vi "Autonomous Independent.vi"() -> ()   [LabVIEW 2020]
doc: "This VI is called when autonomous begins, and will automatically be terminated when autonomous ends. You can carry out timed or sensor driven robot movement independently without needing to return to the caller."
uses:
  <vilib>/Rock Robotics/WPI/Utilities/WPI_GetSetVariantRefNum.vi
  <vilib>/Rock Robotics/Network Tables/NT Read String.vi
  <vilib>/Rock Robotics/Network Tables/NT Write Numeric Array.vi
  Robot Global Data.vi
  <vilib>/addons/control/pid/pid.llb/PID (DBL).vi
  <vilib>/Rock Robotics/Network Tables/NT Write String.vi
  <vilib>/addons/control/pid/NI_PID_pid.lvlib
panel:
  out "Current action":string
  # "Be sure to right-click and choose Data Operations>>Make Current Value default if you want to save the array values with the VI"
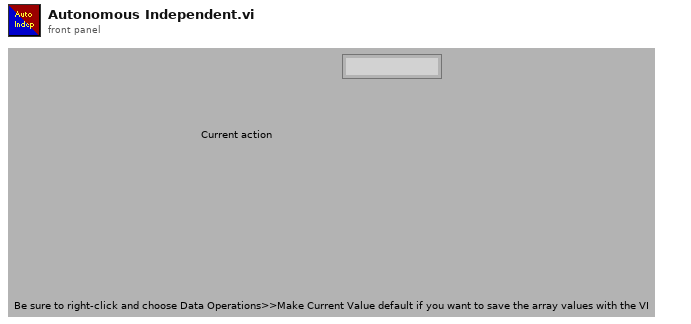
[diagram p1: front panel]
types:
  T1 = typedef "WPI_JoystickDevRef.ctl" = cluster{"Device":T2}
  T2 = typedef "WPI_JoystickDeviceEnum.ctl" = enum16{"USB 0", "USB 1", "USB 2", "USB 3", "USB 4", "USB 5"}
  T3 = cluster{"proportional gain (Kc)":dbl, "integral time (Ti, min)":dbl, "derivative time (Td, min)":dbl}
  T4 = cluster{dbl, "milliseconds to wait":u32, "Name":string}
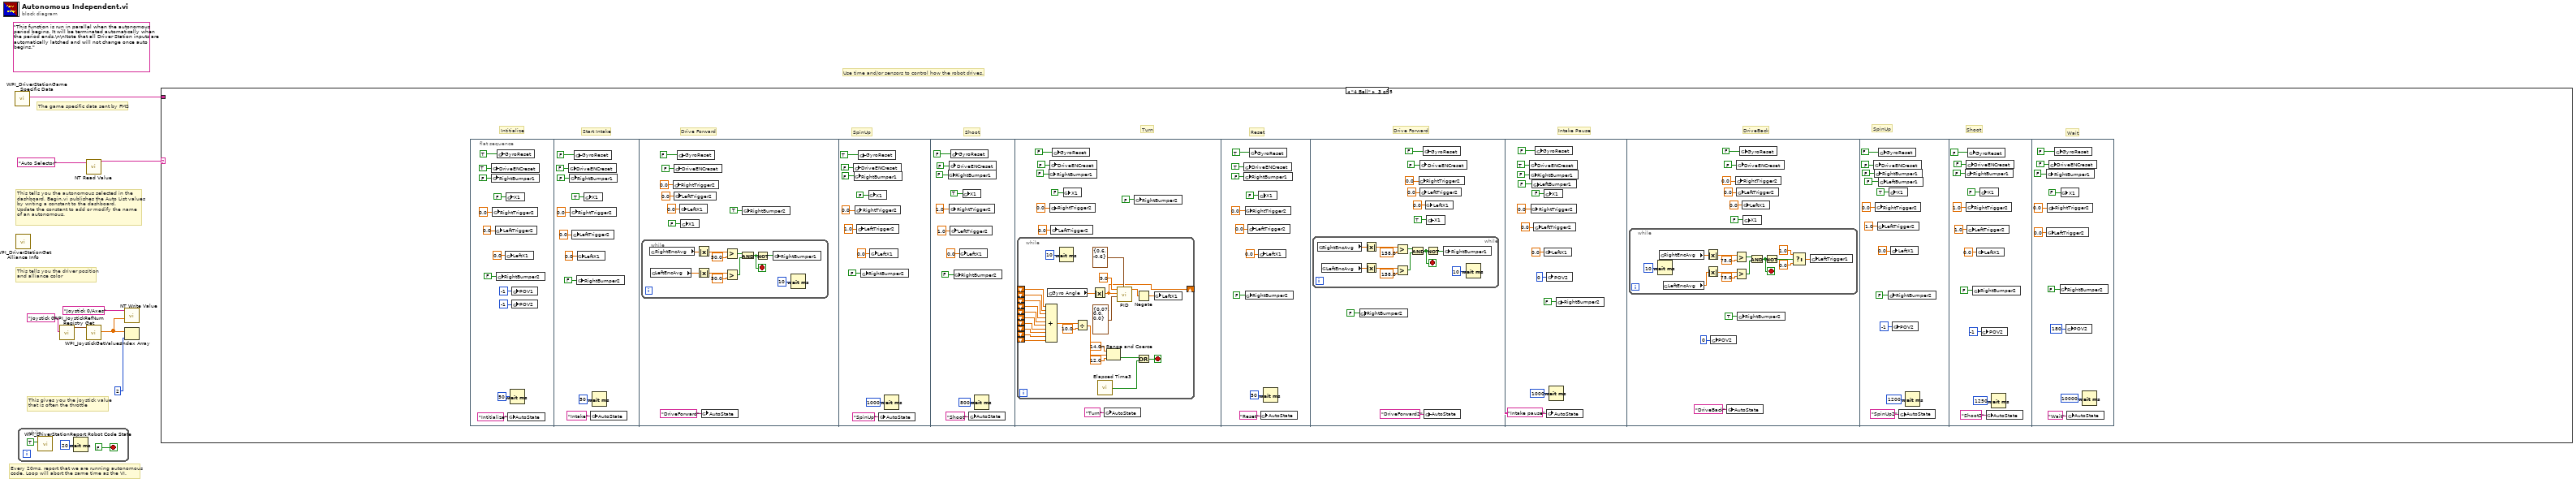
[diagram p0: block diagram]
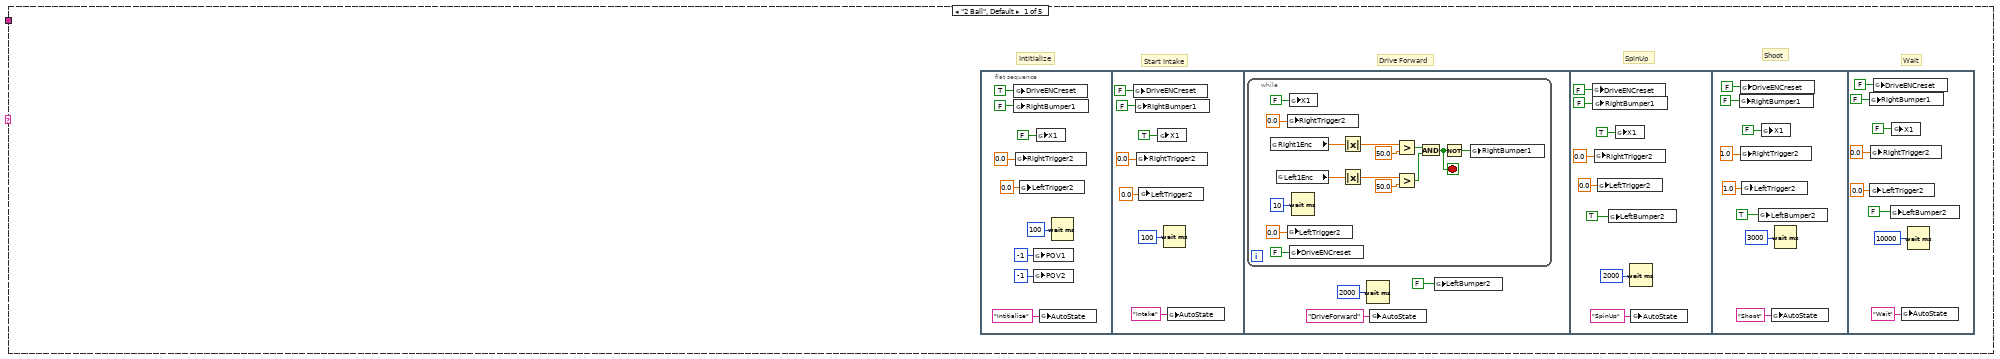
[diagram p2: hidden frame]
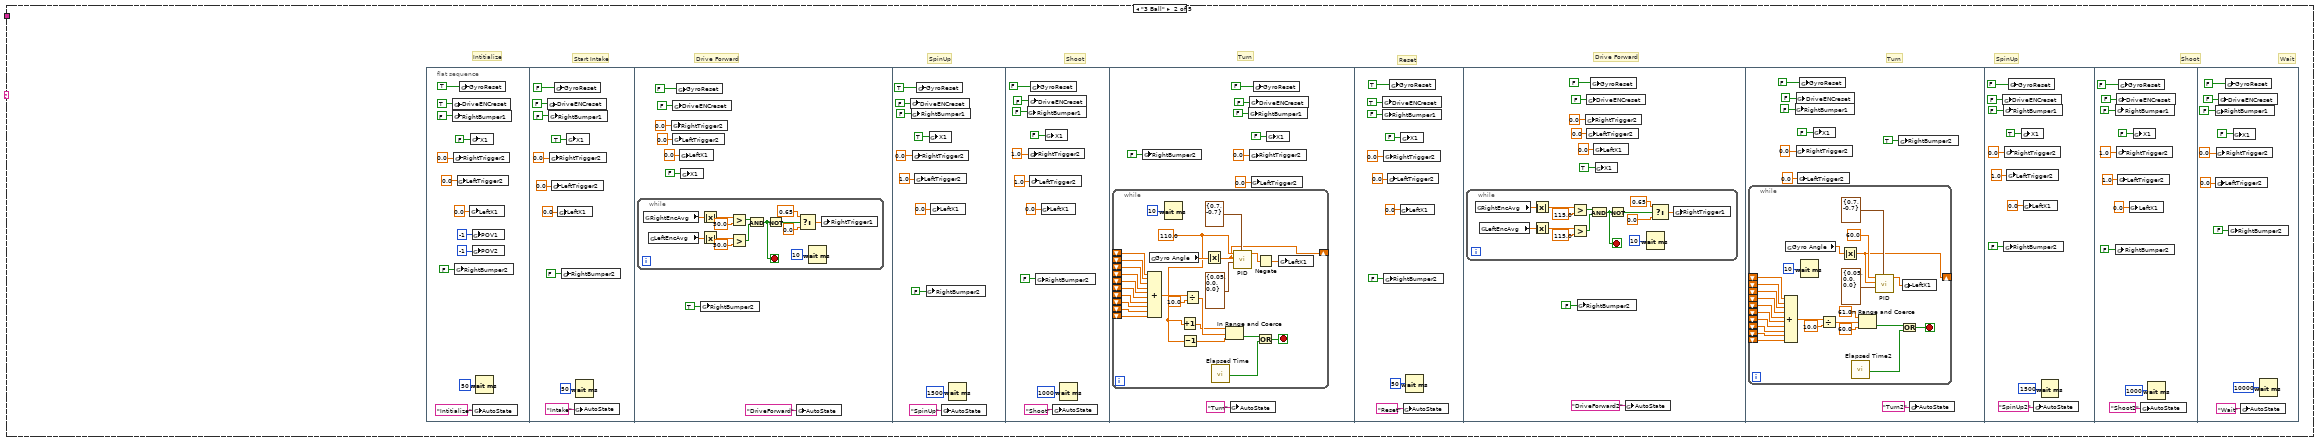
[diagram p3: hidden frame]
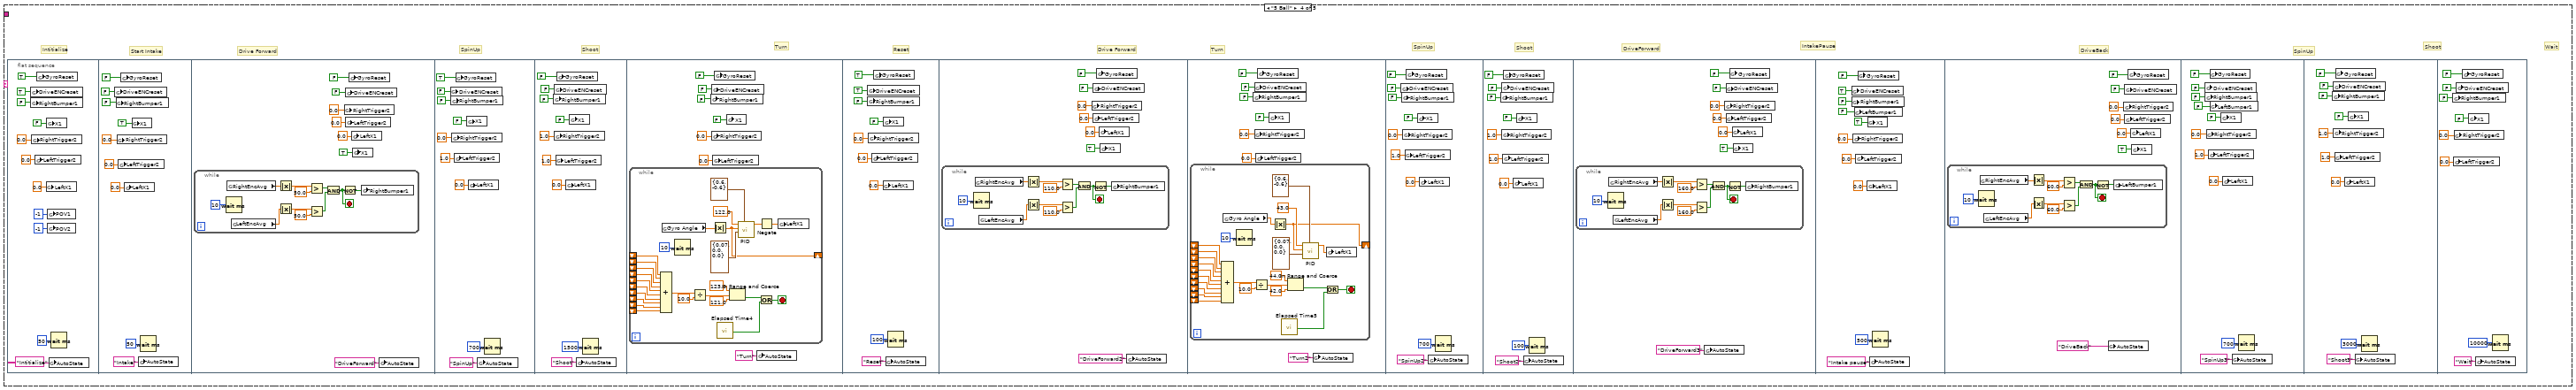
[diagram p4: hidden frame]
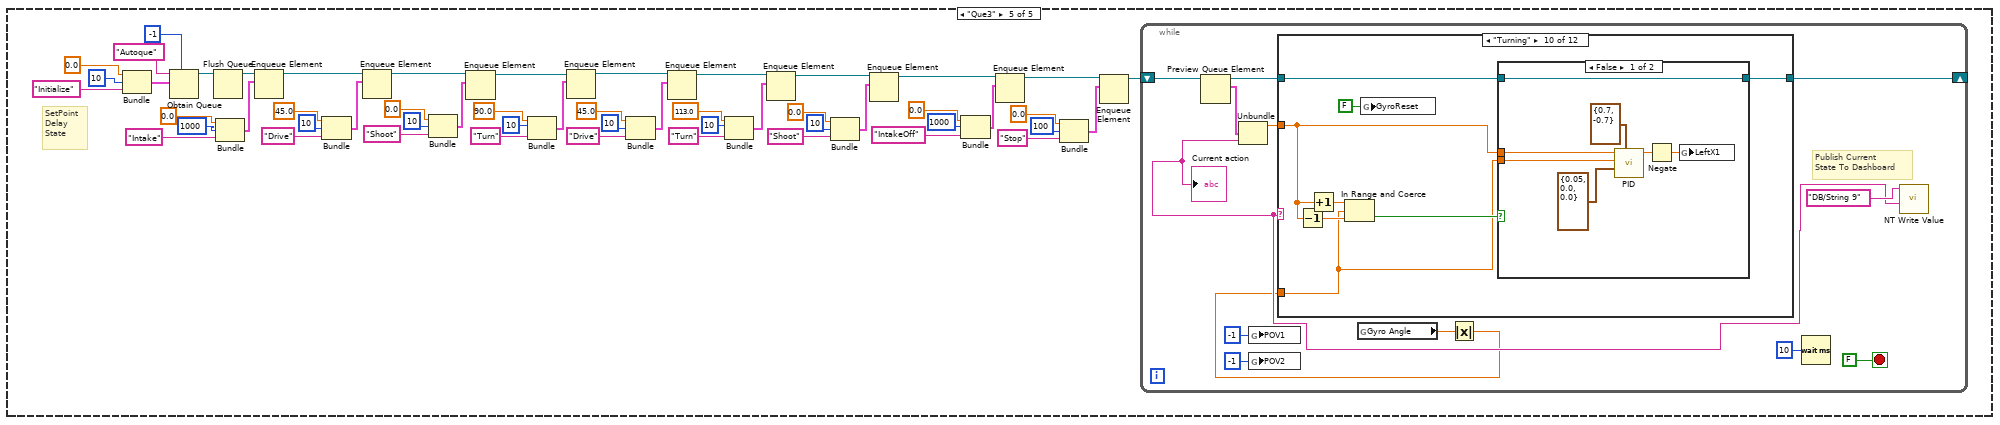
[diagram p5: hidden frame]
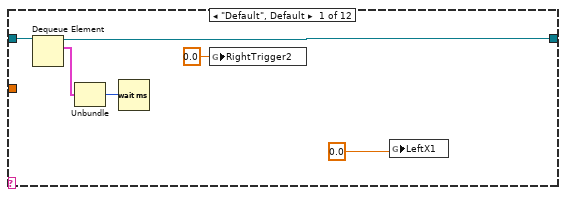
[diagram p6: hidden frame]
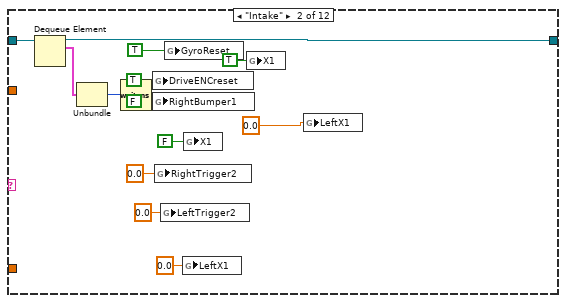
[diagram p7: hidden frame]
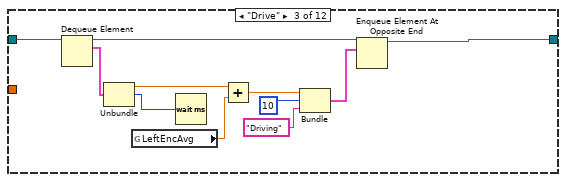
[diagram p8: hidden frame]
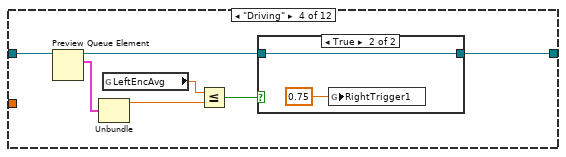
[diagram p9: hidden frame]
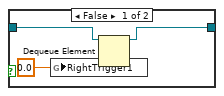
[diagram p10: hidden frame]
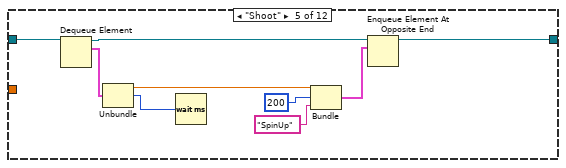
[diagram p11: hidden frame]
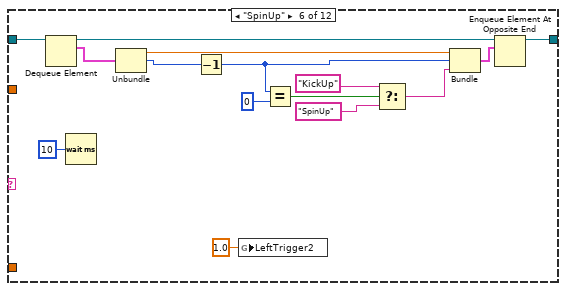
[diagram p12: hidden frame]
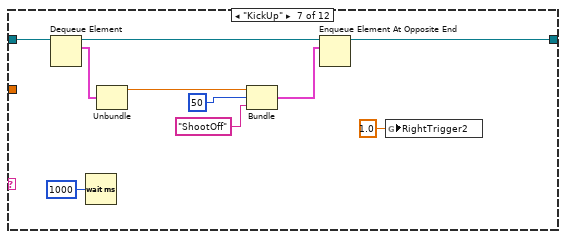
[diagram p13: hidden frame]
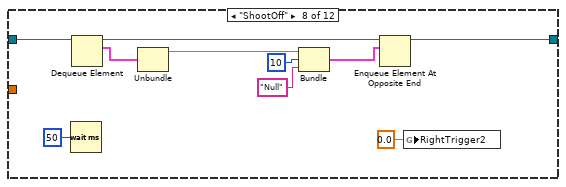
[diagram p14: hidden frame]
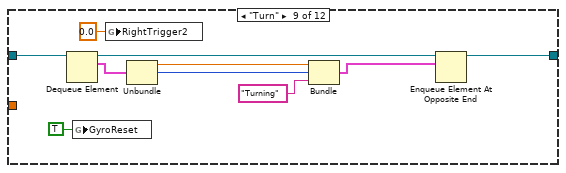
[diagram p15: hidden frame]
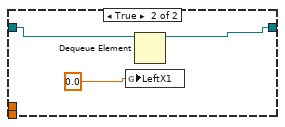
[diagram p16: hidden frame]
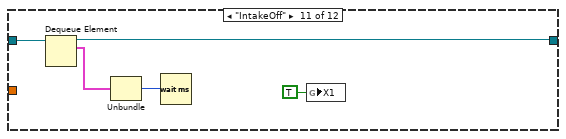
[diagram p17: hidden frame]
diagram:
  (unwired) "This function is run in parallel when the autonomous period begins. It will be terminated automatically when the period ends.\n\nNote that all Driver Station inputs are automatically latched and will not change once auto begins."
  # "The game specific data sent by FMS"
  # "This tells you the autonomous selected in the \ndashboard. Begin.vi publishes the Auto List values\nby writing a constant to the dashboard.\nUpdate the constant to add or modify the name\nof an autonomous."
  # "Every 20ms, report that we are running autonomous\ncode. Loop will abort the same time as the VI."
  # "This gives you the joystick value\nthat is often the throttle"
  # "Use time and/or sensors to control how the robot drives."
  # "This tells you the driver position\nand alliance color"
  n1 = call <vilib>:"WPI_DriverStationGame Specific Data.vi"() -> ("Game Specific Data"=w1:string)  [unwired: 11 in]
  n2 = call <vilib>:"WPI_DriverStationGet Alliance Info.vi"() -> ()  [unwired: 12 out]
  n3 = while {
    stop <- FALSE stop-if-true
    n4 = call <vilib>:"WPI_DriverStationReport Robot Code State.vi"("Autonomous"=TRUE) -> ()  [unwired: 10 in, 1 out]
    n5 = Wait (ms)(milliseconds to wait=u32 20) -> ()  [unwired: 1 out]
  }
  n6 = call <vilib>:"WPI_JoystickRefNum Registry Get.vi"("refnum name"="Joystick 0") -> ("JoystickDevRef"=w7:T1)  [unwired: 1 in, 9 out]
  n7 = call <vilib>:"WPI_JoystickGetValues.vi"("JoystickDevRef"=w7) -> ("Axes"=w3:dbl[])  [unwired: 6 in, 4 out]
  n8 = call-poly <vilib>:"NT Read Value.vi"("Name"="Auto Selector") -> ("String"=w4:string)  [unwired: 9 in, 1 out]
  n9 = call-poly <vilib>:"NT Write Value.vi"("Numeric Array"=w3, "Name"="Joystick 0/Axes") -> ()  [unwired: 9 in, 1 out]
  n10 = Index Array(array=w3, index=2) -> ()  [unwired: 1 out]
  n11 = case shown="\"4 Ball\"" w4 {
    tunnel: w1 -> [_ _ _ _ _]
    frame "2 Ball", Default {
      # "Wait"
      # "Shoot"
      # "SpinUp"
      # "Drive Forward"
      # "Start Intake"
      # "Intitialize"
      n12 = flat-sequence {
        frame #0 {
          n13 = global write "Robot Global Data.vi" "DriveENCreset"(TRUE ("RightBumper1")) -> ()
          n14 = global write "Robot Global Data.vi" "RightBumper1"(FALSE ("RightBumper1")) -> ()
          n15 = global write "Robot Global Data.vi" "RightTrigger2"(0.0 ("RightTrigger2")) -> ()
          n16 = global write "Robot Global Data.vi" "LeftTrigger2"(0.0 ("LeftTrigger2")) -> ()
          n17 = global write "Robot Global Data.vi" "POV1"(i16 -1 ("POV1")) -> ()
          n18 = global write "Robot Global Data.vi" "POV2"(i16 -1 ("POV2")) -> ()
          n19 = global write "Robot Global Data.vi" "X1"(FALSE ("X1")) -> ()
          n20 = global write "Robot Global Data.vi" "AutoState"("Intitialize" ("AutoState")) -> ()
          n21 = Wait (ms)(milliseconds to wait=u32 100) -> ()  [unwired: 1 out]
        }
        frame #1 {
          n22 = global write "Robot Global Data.vi" "DriveENCreset"(FALSE ("RightBumper1")) -> ()
          n23 = global write "Robot Global Data.vi" "RightBumper1"(FALSE ("RightBumper1")) -> ()
          n24 = global write "Robot Global Data.vi" "RightTrigger2"(0.0 ("RightTrigger2")) -> ()
          n25 = global write "Robot Global Data.vi" "LeftTrigger2"(0.0 ("LeftTrigger2")) -> ()
          n26 = global write "Robot Global Data.vi" "X1"(TRUE ("X1")) -> ()
          n27 = Wait (ms)(milliseconds to wait=u32 100) -> ()  [unwired: 1 out]
          n28 = global write "Robot Global Data.vi" "AutoState"("Intake" ("AutoState")) -> ()
        }
        frame #2 {
          n29 = while {
            stop <- w32 stop-if-true
            n30 = global read "Robot Global Data.vi" "Right1Enc"() -> (w43:dbl)
            n31 = global read "Robot Global Data.vi" "Left1Enc"() -> (w42:dbl)
            n32 = global write "Robot Global Data.vi" "RightTrigger2"(0.0 ("RightTrigger2")) -> ()
            n33 = global write "Robot Global Data.vi" "LeftTrigger2"(0.0 ("LeftTrigger2")) -> ()
            n34 = global write "Robot Global Data.vi" "X1"(FALSE ("X1")) -> ()
            n35 = global write "Robot Global Data.vi" "DriveENCreset"(FALSE ("RightBumper1")) -> ()
            n36 = Wait (ms)(milliseconds to wait=u32 10) -> ()  [unwired: 1 out]
            n37 = Absolute Value(x=w43) -> (abs(x)=w35:dbl)
            n38 = Absolute Value(x=w42) -> (abs(x)=w34:dbl)
            n39 = Greater?(x=w35, y=50.0) -> (0:w40:bool)
            n40 = Greater?(x=w34, y=50.0) -> (0:w41:bool)
            n41 = And(x=w40, y=w41) -> (x .and. y?=w32:bool)
            n42 = Not(x=w32) -> (.not. x?=w37:bool)
            n43 = global write "Robot Global Data.vi" "RightBumper1"(w37) -> ()
          }
          n44 = Wait (ms)(milliseconds to wait=u32 2000) -> ()  [unwired: 1 out]
          n45 = global write "Robot Global Data.vi" "AutoState"("DriveForward" ("AutoState")) -> ()
          n46 = global write "Robot Global Data.vi" "LeftBumper2"(FALSE ("RightBumper1")) -> ()
        }
        frame #3 {
          n47 = global write "Robot Global Data.vi" "DriveENCreset"(FALSE ("RightBumper1")) -> ()
          n48 = global write "Robot Global Data.vi" "RightBumper1"(FALSE ("RightBumper1")) -> ()
          n49 = global write "Robot Global Data.vi" "RightTrigger2"(0.0 ("RightTrigger2")) -> ()
          n50 = global write "Robot Global Data.vi" "LeftTrigger2"(0.0 ("LeftTrigger2")) -> ()
          n51 = global write "Robot Global Data.vi" "LeftBumper2"(TRUE ("RightBumper1")) -> ()
          n52 = global write "Robot Global Data.vi" "X1"(TRUE ("X1")) -> ()
          n53 = Wait (ms)(milliseconds to wait=u32 2000) -> ()  [unwired: 1 out]
          n54 = global write "Robot Global Data.vi" "AutoState"("SpinUp" ("AutoState")) -> ()
        }
        frame #4 {
          n55 = global write "Robot Global Data.vi" "RightBumper1"(FALSE ("RightBumper1")) -> ()
          n56 = global write "Robot Global Data.vi" "DriveENCreset"(FALSE ("RightBumper1")) -> ()
          n57 = global write "Robot Global Data.vi" "RightTrigger2"(1.0 ("RightTrigger2")) -> ()
          n58 = global write "Robot Global Data.vi" "LeftTrigger2"(1.0 ("LeftTrigger2")) -> ()
          n59 = global write "Robot Global Data.vi" "LeftBumper2"(TRUE ("RightBumper1")) -> ()
          n60 = global write "Robot Global Data.vi" "X1"(FALSE ("X1")) -> ()
          n61 = global write "Robot Global Data.vi" "AutoState"("Shoot" ("AutoState")) -> ()
          n62 = Wait (ms)(milliseconds to wait=u32 3000) -> ()  [unwired: 1 out]
        }
        frame #5 {
          n63 = global write "Robot Global Data.vi" "RightBumper1"(FALSE ("RightBumper1")) -> ()
          n64 = global write "Robot Global Data.vi" "LeftTrigger2"(0.0 ("LeftTrigger2")) -> ()
          n65 = global write "Robot Global Data.vi" "RightTrigger2"(0.0 ("RightTrigger2")) -> ()
          n66 = global write "Robot Global Data.vi" "DriveENCreset"(FALSE ("RightBumper1")) -> ()
          n67 = global write "Robot Global Data.vi" "LeftBumper2"(FALSE ("RightBumper1")) -> ()
          n68 = global write "Robot Global Data.vi" "X1"(FALSE ("X1")) -> ()
          n69 = global write "Robot Global Data.vi" "AutoState"("Wait" ("AutoState")) -> ()
          n70 = Wait (ms)(milliseconds to wait=u32 10000) -> ()  [unwired: 1 out]
        }
      }
    }
    frame "3 Ball" {
      # "Turn"
      # "Shoot"
      # "SpinUp"
      # "Drive Forward"
      # "Reset"
      # "Turn"
      # "Wait"
      # "Shoot"
      # "SpinUp"
      # "Drive Forward"
      # "Start Intake"
      # "Intitialize"
      n71 = flat-sequence {
        frame #0 {
          n72 = global write "Robot Global Data.vi" "DriveENCreset"(TRUE ("RightBumper1")) -> ()
          n73 = global write "Robot Global Data.vi" "RightBumper1"(FALSE ("RightBumper1")) -> ()
          n74 = global write "Robot Global Data.vi" "RightTrigger2"(0.0 ("RightTrigger2")) -> ()
          n75 = global write "Robot Global Data.vi" "RightBumper2"(FALSE ("RightBumper1")) -> ()
          n76 = global write "Robot Global Data.vi" "LeftTrigger2"(0.0 ("LeftTrigger2")) -> ()
          n77 = global write "Robot Global Data.vi" "GyroReset"(TRUE ("RightBumper1")) -> ()
          n78 = global write "Robot Global Data.vi" "LeftX1"(0.0 ("LeftX1")) -> ()
          n79 = global write "Robot Global Data.vi" "X1"(FALSE ("X1")) -> ()
          n80 = global write "Robot Global Data.vi" "POV1"(i16 -1 ("POV1")) -> ()
          n81 = global write "Robot Global Data.vi" "POV2"(i16 -1 ("POV2")) -> ()
          n82 = global write "Robot Global Data.vi" "AutoState"("Intitialize" ("AutoState")) -> ()
          n83 = Wait (ms)(milliseconds to wait=u32 50) -> ()  [unwired: 1 out]
        }
        frame #1 {
          n84 = global write "Robot Global Data.vi" "DriveENCreset"(FALSE ("RightBumper1")) -> ()
          n85 = global write "Robot Global Data.vi" "RightBumper1"(FALSE ("RightBumper1")) -> ()
          n86 = global write "Robot Global Data.vi" "RightTrigger2"(0.0 ("RightTrigger2")) -> ()
          n87 = global write "Robot Global Data.vi" "LeftTrigger2"(0.0 ("LeftTrigger2")) -> ()
          n88 = global write "Robot Global Data.vi" "GyroReset"(FALSE ("RightBumper1")) -> ()
          n89 = global write "Robot Global Data.vi" "LeftX1"(0.0 ("LeftX1")) -> ()
          n90 = global write "Robot Global Data.vi" "RightBumper2"(FALSE ("RightBumper1")) -> ()
          n91 = global write "Robot Global Data.vi" "X1"(TRUE ("X1")) -> ()
          n92 = global write "Robot Global Data.vi" "AutoState"("Intake" ("AutoState")) -> ()
          n93 = Wait (ms)(milliseconds to wait=u32 50) -> ()  [unwired: 1 out]
        }
        frame #2 {
          n94 = while {
            stop <- w104 stop-if-true
            n95 = global read "Robot Global Data.vi" "RightEncAvg"() -> (w113:dbl)
            n96 = global read "Robot Global Data.vi" "LeftEncAvg"() -> (w112:dbl)
            n97 = Absolute Value(x=w113) -> (abs(x)=w107:dbl)
            n98 = Absolute Value(x=w112) -> (abs(x)=w106:dbl)
            n99 = Greater?(x=w107, y=50.0) -> (0:w110:bool)
            n100 = Greater?(x=w106, y=50.0) -> (0:w111:bool)
            n101 = And(x=w110, y=w111) -> (x .and. y?=w104:bool)
            n102 = Not(x=w104) -> (.not. x?=w103:bool)
            n103 = Select(t=0.65, s=w103, f=0.0) -> (s? t:f=w100:dbl)
            n104 = Wait (ms)(milliseconds to wait=u32 10) -> ()  [unwired: 1 out]
            n105 = global write "Robot Global Data.vi" "RightTrigger1"(w100) -> ()
          }
          n106 = global write "Robot Global Data.vi" "RightTrigger2"(0.0 ("RightTrigger2")) -> ()
          n107 = global write "Robot Global Data.vi" "DriveENCreset"(FALSE ("RightBumper1")) -> ()
          n108 = global write "Robot Global Data.vi" "LeftTrigger2"(0.0 ("LeftTrigger2")) -> ()
          n109 = global write "Robot Global Data.vi" "GyroReset"(FALSE ("RightBumper1")) -> ()
          n110 = global write "Robot Global Data.vi" "LeftX1"(0.0 ("LeftX1")) -> ()
          n111 = global write "Robot Global Data.vi" "X1"(FALSE ("X1")) -> ()
          n112 = global write "Robot Global Data.vi" "RightBumper2"(TRUE ("RightBumper1")) -> ()
          n113 = global write "Robot Global Data.vi" "AutoState"("DriveForward" ("AutoState")) -> ()
        }
        frame #3 {
          n114 = global write "Robot Global Data.vi" "DriveENCreset"(FALSE ("RightBumper1")) -> ()
          n115 = global write "Robot Global Data.vi" "RightBumper1"(FALSE ("RightBumper1")) -> ()
          n116 = global write "Robot Global Data.vi" "RightTrigger2"(0.0 ("RightTrigger2")) -> ()
          n117 = global write "Robot Global Data.vi" "LeftTrigger2"(1.0 ("LeftTrigger2")) -> ()
          n118 = global write "Robot Global Data.vi" "GyroReset"(TRUE ("RightBumper1")) -> ()
          n119 = global write "Robot Global Data.vi" "RightBumper2"(FALSE ("RightBumper1")) -> ()
          n120 = global write "Robot Global Data.vi" "X1"(TRUE ("X1")) -> ()
          n121 = global write "Robot Global Data.vi" "LeftX1"(0.0 ("LeftX1")) -> ()
          n122 = global write "Robot Global Data.vi" "AutoState"("SpinUp" ("AutoState")) -> ()
          n123 = Wait (ms)(milliseconds to wait=u32 1500) -> ()  [unwired: 1 out]
        }
        frame #4 {
          n124 = global write "Robot Global Data.vi" "RightBumper1"(FALSE ("RightBumper1")) -> ()
          n125 = global write "Robot Global Data.vi" "DriveENCreset"(FALSE ("RightBumper1")) -> ()
          n126 = global write "Robot Global Data.vi" "RightTrigger2"(1.0 ("RightTrigger2")) -> ()
          n127 = global write "Robot Global Data.vi" "LeftTrigger2"(1.0 ("LeftTrigger2")) -> ()
          n128 = global write "Robot Global Data.vi" "GyroReset"(FALSE ("RightBumper1")) -> ()
          n129 = global write "Robot Global Data.vi" "RightBumper2"(FALSE ("RightBumper1")) -> ()
          n130 = global write "Robot Global Data.vi" "LeftX1"(0.0 ("LeftX1")) -> ()
          n131 = global write "Robot Global Data.vi" "X1"(FALSE ("X1")) -> ()
          n132 = global write "Robot Global Data.vi" "AutoState"("Shoot" ("AutoState")) -> ()
          n133 = Wait (ms)(milliseconds to wait=u32 1000) -> ()  [unwired: 1 out]
        }
        frame #5 {
          n134 = while {
            shift-right: [w143] -> _
            shift-left: _ -> [w161]
            shift-left: _ -> [w160]
            shift-left: _ -> [w159]
            shift-left: _ -> [w158]
            shift-left: _ -> [w162]
            shift-left: _ -> [w163]
            shift-left: _ -> [w157]
            shift-left: _ -> [w156]
            shift-left: _ -> [w155]
            shift-left: _ -> [w154]
            stop <- w149 stop-if-true
            w144 = 110.0 ("setpoint")
            n135 = Compound Arithmetic op=ADD(w163, w162, w161, w160, w159, w158, w157, w156, w155, w154) -> (w152:dbl)
            n136 = global read "Robot Global Data.vi" "Gyro Angle"() -> (w166:dbl)
            n137 = Wait (ms)(milliseconds to wait=u32 10) -> ()  [unwired: 1 out]
            n138 = Increment(x=w144) -> (x+1=w145:dbl)
            n139 = Decrement(x=w144) -> (x-1=w146:dbl)
            n140 = Divide(x=w152, y=10.0) -> (x/y=w151:dbl)
            n141 = Absolute Value(x=w166) -> (abs(x)=w143:dbl)
            n142 = call "Elapsed Time"() -> ("Time has Elapsed"=w148:bool)  [unwired: 12 in, 7 out]
            n143 = In Range and Coerce(upper limit=w145, x=w151, lower limit=w146) -> (In Range?=w164:bool)  [unwired: 1 out]
            n144 = call-poly <vilib>:"PID.vi"("output range"=cluster{"output high":dbl, "output low":dbl} {"output high"=0.7, "output low"=-0.7}, "PID gains"=T3 {"proportional gain (Kc)"=0.05, "integral time (Ti, min)"=0.0, "derivative time (Td, min)"=0.0}, "process variable"=w143, "setpoint"=w144) -> ("output"=w142:dbl)  [unwired: 6 in, 1 out]
            n145 = Negate(x=w142) -> (-x=w147:dbl)
            n146 = Or(x=w164, y=w148) -> (x .or. y?=w149:bool)
            n147 = global write "Robot Global Data.vi" "LeftX1"(w147) -> ()
          }
          n148 = global write "Robot Global Data.vi" "RightBumper2"(FALSE ("RightBumper1")) -> ()
          n149 = global write "Robot Global Data.vi" "AutoState"("Turn" ("AutoState")) -> ()
          n150 = global write "Robot Global Data.vi" "RightBumper1"(FALSE ("RightBumper1")) -> ()
          n151 = global write "Robot Global Data.vi" "DriveENCreset"(FALSE ("RightBumper1")) -> ()
          n152 = global write "Robot Global Data.vi" "RightTrigger2"(0.0 ("RightTrigger2")) -> ()
          n153 = global write "Robot Global Data.vi" "LeftTrigger2"(0.0 ("LeftTrigger2")) -> ()
          n154 = global write "Robot Global Data.vi" "GyroReset"(FALSE ("RightBumper1")) -> ()
          n155 = global write "Robot Global Data.vi" "X1"(FALSE ("X1")) -> ()
        }
        frame #6 {
          n156 = global write "Robot Global Data.vi" "DriveENCreset"(TRUE ("RightBumper1")) -> ()
          n157 = global write "Robot Global Data.vi" "RightBumper1"(FALSE ("RightBumper1")) -> ()
          n158 = global write "Robot Global Data.vi" "RightTrigger2"(0.0 ("RightTrigger2")) -> ()
          n159 = global write "Robot Global Data.vi" "RightBumper2"(FALSE ("RightBumper1")) -> ()
          n160 = global write "Robot Global Data.vi" "LeftTrigger2"(0.0 ("LeftTrigger2")) -> ()
          n161 = global write "Robot Global Data.vi" "GyroReset"(TRUE ("RightBumper1")) -> ()
          n162 = global write "Robot Global Data.vi" "LeftX1"(0.0 ("LeftX1")) -> ()
          n163 = global write "Robot Global Data.vi" "X1"(FALSE ("X1")) -> ()
          n164 = global write "Robot Global Data.vi" "AutoState"("Reset" ("AutoState")) -> ()
          n165 = Wait (ms)(milliseconds to wait=u32 50) -> ()  [unwired: 1 out]
        }
        frame #7 {
          n166 = while {
            stop <- w190 stop-if-true
            n167 = global read "Robot Global Data.vi" "RightEncAvg"() -> (w199:dbl)
            n168 = global read "Robot Global Data.vi" "LeftEncAvg"() -> (w198:dbl)
            n169 = Absolute Value(x=w199) -> (abs(x)=w193:dbl)
            n170 = Absolute Value(x=w198) -> (abs(x)=w192:dbl)
            n171 = Greater?(x=w193, y=115.0) -> (0:w196:bool)
            n172 = Greater?(x=w192, y=115.0) -> (0:w197:bool)
            n173 = And(x=w196, y=w197) -> (x .and. y?=w190:bool)
            n174 = Not(x=w190) -> (.not. x?=w189:bool)
            n175 = Wait (ms)(milliseconds to wait=u32 10) -> ()  [unwired: 1 out]
            n176 = Select(t=0.65, s=w189, f=0.0) -> (s? t:f=w188:dbl)
            n177 = global write "Robot Global Data.vi" "RightTrigger1"(w188) -> ()
          }
          n178 = global write "Robot Global Data.vi" "RightBumper2"(FALSE ("RightBumper1")) -> ()
          n179 = global write "Robot Global Data.vi" "RightTrigger2"(0.0 ("RightTrigger2")) -> ()
          n180 = global write "Robot Global Data.vi" "DriveENCreset"(FALSE ("RightBumper1")) -> ()
          n181 = global write "Robot Global Data.vi" "LeftTrigger2"(0.0 ("LeftTrigger2")) -> ()
          n182 = global write "Robot Global Data.vi" "GyroReset"(FALSE ("RightBumper1")) -> ()
          n183 = global write "Robot Global Data.vi" "LeftX1"(0.0 ("LeftX1")) -> ()
          n184 = global write "Robot Global Data.vi" "X1"(TRUE ("X1")) -> ()
          n185 = global write "Robot Global Data.vi" "AutoState"("DriveForward2" ("AutoState")) -> ()
        }
        frame #8 {
          n186 = while {
            shift-right: [w208] -> _
            shift-left: _ -> [w222]
            shift-left: _ -> [w221]
            shift-left: _ -> [w220]
            shift-left: _ -> [w219]
            shift-left: _ -> [w223]
            shift-left: _ -> [w224]
            shift-left: _ -> [w218]
            shift-left: _ -> [w217]
            shift-left: _ -> [w216]
            shift-left: _ -> [w215]
            stop <- w210 stop-if-true
            n187 = Compound Arithmetic op=ADD(w224, w223, w222, w221, w220, w219, w218, w217, w216, w215) -> (w213:dbl)
            n188 = global read "Robot Global Data.vi" "Gyro Angle"() -> (w231:dbl)
            n189 = Wait (ms)(milliseconds to wait=u32 10) -> ()  [unwired: 1 out]
            n190 = Divide(x=w213, y=10.0) -> (x/y=w212:dbl)
            n191 = Absolute Value(x=w231) -> (abs(x)=w208:dbl)
            n192 = call "Elapsed Time2"() -> ("Time has Elapsed"=w209:bool)  [unwired: 12 in, 7 out]
            n193 = In Range and Coerce(upper limit=61.0, x=w212, lower limit=60.0) -> (In Range?=w228:bool)  [unwired: 1 out]
            n194 = call-poly <vilib>:"PID.vi"("output range"=cluster{"output high":dbl, "output low":dbl} {"output high"=0.7, "output low"=-0.7}, "PID gains"=T3 {"proportional gain (Kc)"=0.05, "integral time (Ti, min)"=0.0, "derivative time (Td, min)"=0.0}, "process variable"=w208, "setpoint"=60.0) -> ("output"=w225:dbl)  [unwired: 6 in, 1 out]
            n195 = Or(x=w228, y=w209) -> (x .or. y?=w210:bool)
            n196 = global write "Robot Global Data.vi" "LeftX1"(w225) -> ()
          }
          n197 = global write "Robot Global Data.vi" "RightBumper1"(FALSE ("RightBumper1")) -> ()
          n198 = global write "Robot Global Data.vi" "DriveENCreset"(FALSE ("RightBumper1")) -> ()
          n199 = global write "Robot Global Data.vi" "RightTrigger2"(0.0 ("RightTrigger2")) -> ()
          n200 = global write "Robot Global Data.vi" "LeftTrigger2"(0.0 ("LeftTrigger2")) -> ()
          n201 = global write "Robot Global Data.vi" "GyroReset"(FALSE ("RightBumper1")) -> ()
          n202 = global write "Robot Global Data.vi" "X1"(FALSE ("X1")) -> ()
          n203 = global write "Robot Global Data.vi" "RightBumper2"(TRUE ("RightBumper1")) -> ()
          n204 = global write "Robot Global Data.vi" "AutoState"("Turn2" ("AutoState")) -> ()
        }
        frame #9 {
          n205 = global write "Robot Global Data.vi" "DriveENCreset"(FALSE ("RightBumper1")) -> ()
          n206 = global write "Robot Global Data.vi" "RightBumper1"(FALSE ("RightBumper1")) -> ()
          n207 = global write "Robot Global Data.vi" "RightBumper2"(FALSE ("RightBumper1")) -> ()
          n208 = global write "Robot Global Data.vi" "RightTrigger2"(0.0 ("RightTrigger2")) -> ()
          n209 = global write "Robot Global Data.vi" "LeftTrigger2"(1.0 ("LeftTrigger2")) -> ()
          n210 = global write "Robot Global Data.vi" "GyroReset"(FALSE ("RightBumper1")) -> ()
          n211 = global write "Robot Global Data.vi" "X1"(TRUE ("X1")) -> ()
          n212 = global write "Robot Global Data.vi" "LeftX1"(0.0 ("LeftX1")) -> ()
          n213 = global write "Robot Global Data.vi" "AutoState"("SpinUp2" ("AutoState")) -> ()
          n214 = Wait (ms)(milliseconds to wait=u32 1500) -> ()  [unwired: 1 out]
        }
        frame #10 {
          n215 = global write "Robot Global Data.vi" "RightBumper1"(FALSE ("RightBumper1")) -> ()
          n216 = global write "Robot Global Data.vi" "RightBumper2"(FALSE ("RightBumper1")) -> ()
          n217 = global write "Robot Global Data.vi" "DriveENCreset"(FALSE ("RightBumper1")) -> ()
          n218 = global write "Robot Global Data.vi" "RightTrigger2"(1.0 ("RightTrigger2")) -> ()
          n219 = global write "Robot Global Data.vi" "LeftTrigger2"(1.0 ("LeftTrigger2")) -> ()
          n220 = global write "Robot Global Data.vi" "GyroReset"(FALSE ("RightBumper1")) -> ()
          n221 = global write "Robot Global Data.vi" "LeftX1"(0.0 ("LeftX1")) -> ()
          n222 = global write "Robot Global Data.vi" "X1"(FALSE ("X1")) -> ()
          n223 = global write "Robot Global Data.vi" "AutoState"("Shoot2" ("AutoState")) -> ()
          n224 = Wait (ms)(milliseconds to wait=u32 1000) -> ()  [unwired: 1 out]
        }
        frame #11 {
          n225 = global write "Robot Global Data.vi" "RightBumper1"(FALSE ("RightBumper1")) -> ()
          n226 = global write "Robot Global Data.vi" "LeftTrigger2"(0.0 ("LeftTrigger2")) -> ()
          n227 = global write "Robot Global Data.vi" "RightTrigger2"(0.0 ("RightTrigger2")) -> ()
          n228 = global write "Robot Global Data.vi" "DriveENCreset"(FALSE ("RightBumper1")) -> ()
          n229 = global write "Robot Global Data.vi" "GyroReset"(FALSE ("RightBumper1")) -> ()
          n230 = global write "Robot Global Data.vi" "RightBumper2"(FALSE ("RightBumper1")) -> ()
          n231 = global write "Robot Global Data.vi" "X1"(FALSE ("X1")) -> ()
          n232 = global write "Robot Global Data.vi" "AutoState"("Wait" ("AutoState")) -> ()
          n233 = Wait (ms)(milliseconds to wait=u32 10000) -> ()  [unwired: 1 out]
        }
      }
    }
    frame "4 Ball" {
      # "Intake Pause"
      # "DriveBack"
      # "Shoot"
      # "SpinUp"
      # "Drive Forward"
      # "Reset"
      # "Turn"
      # "Wait"
      # "Shoot"
      # "SpinUp"
      # "Drive Forward"
      # "Start Intake"
      # "Intitialize"
      n234 = flat-sequence {
        frame #0 {
          n235 = global write "Robot Global Data.vi" "DriveENCreset"(TRUE ("RightBumper1")) -> ()
          n236 = global write "Robot Global Data.vi" "RightBumper1"(FALSE ("RightBumper1")) -> ()
          n237 = global write "Robot Global Data.vi" "RightTrigger2"(0.0 ("RightTrigger2")) -> ()
          n238 = global write "Robot Global Data.vi" "LeftTrigger2"(0.0 ("LeftTrigger2")) -> ()
          n239 = global write "Robot Global Data.vi" "RightBumper2"(FALSE ("RightBumper1")) -> ()
          n240 = global write "Robot Global Data.vi" "GyroReset"(TRUE ("RightBumper1")) -> ()
          n241 = global write "Robot Global Data.vi" "LeftX1"(0.0 ("LeftX1")) -> ()
          n242 = global write "Robot Global Data.vi" "X1"(FALSE ("X1")) -> ()
          n243 = global write "Robot Global Data.vi" "AutoState"("Intitialize" ("AutoState")) -> ()
          n244 = Wait (ms)(milliseconds to wait=u32 50) -> ()  [unwired: 1 out]
          n245 = global write "Robot Global Data.vi" "POV1"(i16 -1 ("POV1")) -> ()
          n246 = global write "Robot Global Data.vi" "POV2"(i16 -1 ("POV2")) -> ()
        }
        frame #1 {
          n247 = global write "Robot Global Data.vi" "DriveENCreset"(FALSE ("RightBumper1")) -> ()
          n248 = global write "Robot Global Data.vi" "RightBumper1"(FALSE ("RightBumper1")) -> ()
          n249 = global write "Robot Global Data.vi" "RightTrigger2"(0.0 ("RightTrigger2")) -> ()
          n250 = global write "Robot Global Data.vi" "LeftTrigger2"(0.0 ("LeftTrigger2")) -> ()
          n251 = global write "Robot Global Data.vi" "GyroReset"(FALSE ("RightBumper1")) -> ()
          n252 = global write "Robot Global Data.vi" "RightBumper2"(FALSE ("RightBumper1")) -> ()
          n253 = global write "Robot Global Data.vi" "LeftX1"(0.0 ("LeftX1")) -> ()
          n254 = global write "Robot Global Data.vi" "X1"(TRUE ("X1")) -> ()
          n255 = global write "Robot Global Data.vi" "AutoState"("Intake" ("AutoState")) -> ()
          n256 = Wait (ms)(milliseconds to wait=u32 50) -> ()  [unwired: 1 out]
        }
        frame #2 {
          n257 = while {
            stop <- w292 stop-if-true
            n258 = global read "Robot Global Data.vi" "RightEncAvg"() -> (w302:dbl)
            n259 = global read "Robot Global Data.vi" "LeftEncAvg"() -> (w301:dbl)
            n260 = Absolute Value(x=w302) -> (abs(x)=w295:dbl)
            n261 = Absolute Value(x=w301) -> (abs(x)=w294:dbl)
            n262 = Greater?(x=w295, y=50.0) -> (0:w299:bool)
            n263 = Greater?(x=w294, y=50.0) -> (0:w300:bool)
            n264 = And(x=w299, y=w300) -> (x .and. y?=w292:bool)
            n265 = Not(x=w292) -> (.not. x?=w296:bool)
            n266 = global write "Robot Global Data.vi" "RightBumper1"(w296) -> ()
            n267 = Wait (ms)(milliseconds to wait=u32 10) -> ()  [unwired: 1 out]
          }
          n268 = global write "Robot Global Data.vi" "RightTrigger2"(0.0 ("RightTrigger2")) -> ()
          n269 = global write "Robot Global Data.vi" "DriveENCreset"(FALSE ("RightBumper1")) -> ()
          n270 = global write "Robot Global Data.vi" "LeftTrigger2"(0.0 ("LeftTrigger2")) -> ()
          n271 = global write "Robot Global Data.vi" "GyroReset"(FALSE ("RightBumper1")) -> ()
          n272 = global write "Robot Global Data.vi" "LeftX1"(0.0 ("LeftX1")) -> ()
          n273 = global write "Robot Global Data.vi" "X1"(FALSE ("X1")) -> ()
          n274 = global write "Robot Global Data.vi" "AutoState"("DriveForward" ("AutoState")) -> ()
          n275 = global write "Robot Global Data.vi" "RightBumper2"(TRUE ("RightBumper1")) -> ()
        }
        frame #3 {
          n276 = global write "Robot Global Data.vi" "DriveENCreset"(FALSE ("RightBumper1")) -> ()
          n277 = global write "Robot Global Data.vi" "RightBumper1"(FALSE ("RightBumper1")) -> ()
          n278 = global write "Robot Global Data.vi" "RightTrigger2"(0.0 ("RightTrigger2")) -> ()
          n279 = global write "Robot Global Data.vi" "LeftTrigger2"(1.0 ("LeftTrigger2")) -> ()
          n280 = global write "Robot Global Data.vi" "GyroReset"(TRUE ("RightBumper1")) -> ()
          n281 = global write "Robot Global Data.vi" "RightBumper2"(FALSE ("RightBumper1")) -> ()
          n282 = global write "Robot Global Data.vi" "X1"(FALSE ("X1")) -> ()
          n283 = global write "Robot Global Data.vi" "LeftX1"(0.0 ("LeftX1")) -> ()
          n284 = global write "Robot Global Data.vi" "AutoState"("SpinUp" ("AutoState")) -> ()
          n285 = Wait (ms)(milliseconds to wait=u32 1000) -> ()  [unwired: 1 out]
        }
        frame #4 {
          n286 = global write "Robot Global Data.vi" "RightBumper1"(FALSE ("RightBumper1")) -> ()
          n287 = global write "Robot Global Data.vi" "DriveENCreset"(FALSE ("RightBumper1")) -> ()
          n288 = global write "Robot Global Data.vi" "RightTrigger2"(1.0 ("RightTrigger2")) -> ()
          n289 = global write "Robot Global Data.vi" "LeftTrigger2"(1.0 ("LeftTrigger2")) -> ()
          n290 = global write "Robot Global Data.vi" "GyroReset"(FALSE ("RightBumper1")) -> ()
          n291 = global write "Robot Global Data.vi" "RightBumper2"(FALSE ("RightBumper1")) -> ()
          n292 = global write "Robot Global Data.vi" "LeftX1"(0.0 ("LeftX1")) -> ()
          n293 = global write "Robot Global Data.vi" "X1"(TRUE ("X1")) -> ()
          n294 = global write "Robot Global Data.vi" "AutoState"("Shoot" ("AutoState")) -> ()
          n295 = Wait (ms)(milliseconds to wait=u32 800) -> ()  [unwired: 1 out]
        }
        frame #5 {
          n296 = while {
            shift-right: [w331] -> _
            shift-left: _ -> [w346]
            shift-left: _ -> [w345]
            shift-left: _ -> [w344]
            shift-left: _ -> [w343]
            shift-left: _ -> [w347]
            shift-left: _ -> [w348]
            shift-left: _ -> [w342]
            shift-left: _ -> [w341]
            shift-left: _ -> [w340]
            shift-left: _ -> [w339]
            stop <- w334 stop-if-true
            n297 = Compound Arithmetic op=ADD(w348, w347, w346, w345, w344, w343, w342, w341, w340, w339) -> (w337:dbl)
            n298 = global read "Robot Global Data.vi" "Gyro Angle"() -> (w355:dbl)
            n299 = Wait (ms)(milliseconds to wait=u32 10) -> ()  [unwired: 1 out]
            n300 = Divide(x=w337, y=10.0) -> (x/y=w336:dbl)
            n301 = Absolute Value(x=w355) -> (abs(x)=w331:dbl)
            n302 = call "Elapsed Time3"() -> ("Time has Elapsed"=w333:bool)  [unwired: 12 in, 7 out]
            n303 = In Range and Coerce(upper limit=14.0, x=w336, lower limit=12.0) -> (In Range?=w352:bool)  [unwired: 1 out]
            n304 = call-poly <vilib>:"PID.vi"("output range"=cluster{"output high":dbl, "output low":dbl} {"output high"=0.6, "output low"=-0.6}, "PID gains"=T3 {"proportional gain (Kc)"=0.07, "integral time (Ti, min)"=0.0, "derivative time (Td, min)"=0.0}, "process variable"=w331, "setpoint"=9.0) -> ("output"=w349:dbl)  [unwired: 6 in, 1 out]
            n305 = Negate(x=w349) -> (-x=w332:dbl)
            n306 = Or(x=w352, y=w333) -> (x .or. y?=w334:bool)
            n307 = global write "Robot Global Data.vi" "LeftX1"(w332) -> ()
          }
          n308 = global write "Robot Global Data.vi" "RightBumper1"(FALSE ("RightBumper1")) -> ()
          n309 = global write "Robot Global Data.vi" "DriveENCreset"(FALSE ("RightBumper1")) -> ()
          n310 = global write "Robot Global Data.vi" "RightTrigger2"(0.0 ("RightTrigger2")) -> ()
          n311 = global write "Robot Global Data.vi" "LeftTrigger2"(0.0 ("LeftTrigger2")) -> ()
          n312 = global write "Robot Global Data.vi" "GyroReset"(FALSE ("RightBumper1")) -> ()
          n313 = global write "Robot Global Data.vi" "X1"(FALSE ("X1")) -> ()
          n314 = global write "Robot Global Data.vi" "AutoState"("Turn" ("AutoState")) -> ()
          n315 = global write "Robot Global Data.vi" "RightBumper2"(FALSE ("RightBumper1")) -> ()
        }
        frame #6 {
          n316 = global write "Robot Global Data.vi" "DriveENCreset"(TRUE ("RightBumper1")) -> ()
          n317 = global write "Robot Global Data.vi" "RightBumper1"(FALSE ("RightBumper1")) -> ()
          n318 = global write "Robot Global Data.vi" "RightTrigger2"(0.0 ("RightTrigger2")) -> ()
          n319 = global write "Robot Global Data.vi" "RightBumper2"(FALSE ("RightBumper1")) -> ()
          n320 = global write "Robot Global Data.vi" "LeftTrigger2"(0.0 ("LeftTrigger2")) -> ()
          n321 = global write "Robot Global Data.vi" "GyroReset"(TRUE ("RightBumper1")) -> ()
          n322 = global write "Robot Global Data.vi" "LeftX1"(0.0 ("LeftX1")) -> ()
          n323 = global write "Robot Global Data.vi" "X1"(FALSE ("X1")) -> ()
          n324 = global write "Robot Global Data.vi" "AutoState"("Reset" ("AutoState")) -> ()
          n325 = Wait (ms)(milliseconds to wait=u32 50) -> ()  [unwired: 1 out]
        }
        frame #7 {
          n326 = while {
            stop <- w375 stop-if-true
            n327 = global read "Robot Global Data.vi" "RightEncAvg"() -> (w385:dbl)
            n328 = global read "Robot Global Data.vi" "LeftEncAvg"() -> (w384:dbl)
            n329 = Absolute Value(x=w385) -> (abs(x)=w378:dbl)
            n330 = Absolute Value(x=w384) -> (abs(x)=w377:dbl)
            n331 = Greater?(x=w378, y=158.0) -> (0:w382:bool)
            n332 = Greater?(x=w377, y=158.0) -> (0:w383:bool)
            n333 = And(x=w382, y=w383) -> (x .and. y?=w375:bool)
            n334 = Not(x=w375) -> (.not. x?=w379:bool)
            n335 = global write "Robot Global Data.vi" "RightBumper1"(w379) -> ()
            n336 = Wait (ms)(milliseconds to wait=u32 10) -> ()  [unwired: 1 out]
          }
          n337 = global write "Robot Global Data.vi" "RightBumper2"(FALSE ("RightBumper1")) -> ()
          n338 = global write "Robot Global Data.vi" "RightTrigger2"(0.0 ("RightTrigger2")) -> ()
          n339 = global write "Robot Global Data.vi" "DriveENCreset"(FALSE ("RightBumper1")) -> ()
          n340 = global write "Robot Global Data.vi" "LeftTrigger2"(0.0 ("LeftTrigger2")) -> ()
          n341 = global write "Robot Global Data.vi" "GyroReset"(FALSE ("RightBumper1")) -> ()
          n342 = global write "Robot Global Data.vi" "AutoState"("DriveForward2" ("AutoState")) -> ()
          n343 = global write "Robot Global Data.vi" "LeftX1"(0.0 ("LeftX1")) -> ()
          n344 = global write "Robot Global Data.vi" "X1"(TRUE ("X1")) -> ()
        }
        frame #8 {
          n345 = global write "Robot Global Data.vi" "DriveENCreset"(TRUE ("RightBumper1")) -> ()
          n346 = global write "Robot Global Data.vi" "RightBumper1"(FALSE ("RightBumper1")) -> ()
          n347 = global write "Robot Global Data.vi" "RightTrigger2"(0.0 ("RightTrigger2")) -> ()
          n348 = global write "Robot Global Data.vi" "LeftBumper1"(FALSE ("RightBumper1")) -> ()
          n349 = global write "Robot Global Data.vi" "LeftTrigger2"(0.0 ("LeftTrigger2")) -> ()
          n350 = global write "Robot Global Data.vi" "GyroReset"(FALSE ("RightBumper1")) -> ()
          n351 = global write "Robot Global Data.vi" "LeftX1"(0.0 ("LeftX1")) -> ()
          n352 = global write "Robot Global Data.vi" "X1"(FALSE ("X1")) -> ()
          n353 = global write "Robot Global Data.vi" "POV2"(i16 0 ("POV2")) -> ()
          n354 = global write "Robot Global Data.vi" "AutoState"("Intake pause" ("AutoState")) -> ()
          n355 = Wait (ms)(milliseconds to wait=u32 1000) -> ()  [unwired: 1 out]
          n356 = global write "Robot Global Data.vi" "RightBumper2"(FALSE ("RightBumper1")) -> ()
        }
        frame #9 {
          n357 = while {
            stop <- w411 stop-if-true
            n358 = Wait (ms)(milliseconds to wait=u32 10) -> ()  [unwired: 1 out]
            n359 = global read "Robot Global Data.vi" "RightEncAvg"() -> (w420:dbl)
            n360 = global read "Robot Global Data.vi" "LeftEncAvg"() -> (w419:dbl)
            n361 = Absolute Value(x=w420) -> (abs(x)=w414:dbl)
            n362 = Absolute Value(x=w419) -> (abs(x)=w413:dbl)
            n363 = Greater?(x=w414, y=75.0) -> (0:w417:bool)
            n364 = Greater?(x=w413, y=75.0) -> (0:w418:bool)
            n365 = And(x=w417, y=w418) -> (x .and. y?=w411:bool)
            n366 = Not(x=w411) -> (.not. x?=w410:bool)
            n367 = Select(t=1.0, s=w410, f=0.0) -> (s? t:f=w409:dbl)
            n368 = global write "Robot Global Data.vi" "LeftTrigger1"(w409) -> ()
          }
          n369 = global write "Robot Global Data.vi" "POV2"(i16 0 ("POV2")) -> ()
          n370 = global write "Robot Global Data.vi" "AutoState"("DriveBack" ("AutoState")) -> ()
          n371 = global write "Robot Global Data.vi" "RightTrigger2"(0.0 ("RightTrigger2")) -> ()
          n372 = global write "Robot Global Data.vi" "DriveENCreset"(FALSE ("RightBumper1")) -> ()
          n373 = global write "Robot Global Data.vi" "LeftTrigger2"(0.0 ("LeftTrigger2")) -> ()
          n374 = global write "Robot Global Data.vi" "RightBumper2"(TRUE ("RightBumper1")) -> ()
          n375 = global write "Robot Global Data.vi" "GyroReset"(FALSE ("RightBumper1")) -> ()
          n376 = global write "Robot Global Data.vi" "LeftX1"(0.0 ("LeftX1")) -> ()
          n377 = global write "Robot Global Data.vi" "X1"(FALSE ("X1")) -> ()
        }
        frame #10 {
          n378 = global write "Robot Global Data.vi" "DriveENCreset"(FALSE ("RightBumper1")) -> ()
          n379 = global write "Robot Global Data.vi" "RightBumper1"(FALSE ("RightBumper1")) -> ()
          n380 = global write "Robot Global Data.vi" "RightTrigger2"(0.0 ("RightTrigger2")) -> ()
          n381 = global write "Robot Global Data.vi" "LeftTrigger2"(1.0 ("LeftTrigger2")) -> ()
          n382 = global write "Robot Global Data.vi" "GyroReset"(FALSE ("RightBumper1")) -> ()
          n383 = global write "Robot Global Data.vi" "LeftBumper1"(FALSE ("RightBumper1")) -> ()
          n384 = global write "Robot Global Data.vi" "RightBumper2"(FALSE ("RightBumper1")) -> ()
          n385 = global write "Robot Global Data.vi" "X1"(TRUE ("X1")) -> ()
          n386 = global write "Robot Global Data.vi" "LeftX1"(0.0 ("LeftX1")) -> ()
          n387 = global write "Robot Global Data.vi" "POV2"(i16 -1 ("POV2")) -> ()
          n388 = global write "Robot Global Data.vi" "AutoState"("SpinUp2" ("AutoState")) -> ()
          n389 = Wait (ms)(milliseconds to wait=u32 1200) -> ()  [unwired: 1 out]
        }
        frame #11 {
          n390 = global write "Robot Global Data.vi" "RightBumper1"(FALSE ("RightBumper1")) -> ()
          n391 = global write "Robot Global Data.vi" "DriveENCreset"(FALSE ("RightBumper1")) -> ()
          n392 = global write "Robot Global Data.vi" "RightTrigger2"(1.0 ("RightTrigger2")) -> ()
          n393 = global write "Robot Global Data.vi" "LeftTrigger2"(1.0 ("LeftTrigger2")) -> ()
          n394 = global write "Robot Global Data.vi" "GyroReset"(FALSE ("RightBumper1")) -> ()
          n395 = global write "Robot Global Data.vi" "RightBumper2"(FALSE ("RightBumper1")) -> ()
          n396 = global write "Robot Global Data.vi" "LeftX1"(0.0 ("LeftX1")) -> ()
          n397 = global write "Robot Global Data.vi" "X1"(FALSE ("X1")) -> ()
          n398 = global write "Robot Global Data.vi" "POV2"(i16 -1 ("POV2")) -> ()
          n399 = global write "Robot Global Data.vi" "AutoState"("Shoot2" ("AutoState")) -> ()
          n400 = Wait (ms)(milliseconds to wait=u32 1250) -> ()  [unwired: 1 out]
        }
        frame #12 {
          n401 = global write "Robot Global Data.vi" "RightBumper1"(FALSE ("RightBumper1")) -> ()
          n402 = global write "Robot Global Data.vi" "LeftTrigger2"(0.0 ("LeftTrigger2")) -> ()
          n403 = global write "Robot Global Data.vi" "RightTrigger2"(0.0 ("RightTrigger2")) -> ()
          n404 = global write "Robot Global Data.vi" "DriveENCreset"(FALSE ("RightBumper1")) -> ()
          n405 = global write "Robot Global Data.vi" "GyroReset"(FALSE ("RightBumper1")) -> ()
          n406 = global write "Robot Global Data.vi" "RightBumper2"(FALSE ("RightBumper1")) -> ()
          n407 = global write "Robot Global Data.vi" "X1"(FALSE ("X1")) -> ()
          n408 = global write "Robot Global Data.vi" "POV2"(i16 180 ("POV2")) -> ()
          n409 = global write "Robot Global Data.vi" "AutoState"("Wait" ("AutoState")) -> ()
          n410 = Wait (ms)(milliseconds to wait=u32 10000) -> ()  [unwired: 1 out]
        }
      }
    }
    frame "5 Ball" {
      # "Shoot"
      # "SpinUp"
      # "DriveBack"
      # "IntakePause"
      # "DriveForward"
      # "Turn"
      # "Shoot"
      # "SpinUp"
      # "Drive Forward"
      # "Reset"
      # "Turn"
      # "Wait"
      # "Shoot"
      # "SpinUp"
      # "Drive Forward"
      # "Start Intake"
      # "Intitialize"
      n411 = flat-sequence {
        frame #0 {
          n412 = global write "Robot Global Data.vi" "DriveENCreset"(TRUE ("RightBumper1")) -> ()
          n413 = global write "Robot Global Data.vi" "RightBumper1"(FALSE ("RightBumper1")) -> ()
          n414 = global write "Robot Global Data.vi" "RightTrigger2"(0.0 ("RightTrigger2")) -> ()
          n415 = global write "Robot Global Data.vi" "LeftTrigger2"(0.0 ("LeftTrigger2")) -> ()
          n416 = global write "Robot Global Data.vi" "GyroReset"(TRUE ("RightBumper1")) -> ()
          n417 = global write "Robot Global Data.vi" "LeftX1"(0.0 ("LeftX1")) -> ()
          n418 = global write "Robot Global Data.vi" "X1"(FALSE ("X1")) -> ()
          n419 = global write "Robot Global Data.vi" "POV1"(i16 -1 ("POV1")) -> ()
          n420 = global write "Robot Global Data.vi" "POV2"(i16 -1 ("POV2")) -> ()
          n421 = global write "Robot Global Data.vi" "AutoState"("Intitialize" ("AutoState")) -> ()
          n422 = Wait (ms)(milliseconds to wait=u32 50) -> ()  [unwired: 1 out]
        }
        frame #1 {
          n423 = global write "Robot Global Data.vi" "DriveENCreset"(FALSE ("RightBumper1")) -> ()
          n424 = global write "Robot Global Data.vi" "RightBumper1"(FALSE ("RightBumper1")) -> ()
          n425 = global write "Robot Global Data.vi" "RightTrigger2"(0.0 ("RightTrigger2")) -> ()
          n426 = global write "Robot Global Data.vi" "LeftTrigger2"(0.0 ("LeftTrigger2")) -> ()
          n427 = global write "Robot Global Data.vi" "GyroReset"(FALSE ("RightBumper1")) -> ()
          n428 = global write "Robot Global Data.vi" "LeftX1"(0.0 ("LeftX1")) -> ()
          n429 = global write "Robot Global Data.vi" "X1"(TRUE ("X1")) -> ()
          n430 = global write "Robot Global Data.vi" "AutoState"("Intake" ("AutoState")) -> ()
          n431 = Wait (ms)(milliseconds to wait=u32 50) -> ()  [unwired: 1 out]
        }
        frame #2 {
          n432 = while {
            stop <- w481 stop-if-true
            n433 = Wait (ms)(milliseconds to wait=u32 10) -> ()  [unwired: 1 out]
            n434 = global read "Robot Global Data.vi" "RightEncAvg"() -> (w491:dbl)
            n435 = global read "Robot Global Data.vi" "LeftEncAvg"() -> (w490:dbl)
            n436 = Absolute Value(x=w491) -> (abs(x)=w484:dbl)
            n437 = Absolute Value(x=w490) -> (abs(x)=w483:dbl)
            n438 = Greater?(x=w484, y=50.0) -> (0:w488:bool)
            n439 = Greater?(x=w483, y=50.0) -> (0:w489:bool)
            n440 = And(x=w488, y=w489) -> (x .and. y?=w481:bool)
            n441 = Not(x=w481) -> (.not. x?=w485:bool)
            n442 = global write "Robot Global Data.vi" "RightBumper1"(w485) -> ()
          }
          n443 = global write "Robot Global Data.vi" "RightTrigger2"(0.0 ("RightTrigger2")) -> ()
          n444 = global write "Robot Global Data.vi" "DriveENCreset"(FALSE ("RightBumper1")) -> ()
          n445 = global write "Robot Global Data.vi" "LeftTrigger2"(0.0 ("LeftTrigger2")) -> ()
          n446 = global write "Robot Global Data.vi" "GyroReset"(FALSE ("RightBumper1")) -> ()
          n447 = global write "Robot Global Data.vi" "LeftX1"(0.0 ("LeftX1")) -> ()
          n448 = global write "Robot Global Data.vi" "X1"(TRUE ("X1")) -> ()
          n449 = global write "Robot Global Data.vi" "AutoState"("DriveForward" ("AutoState")) -> ()
        }
        frame #3 {
          n450 = global write "Robot Global Data.vi" "DriveENCreset"(FALSE ("RightBumper1")) -> ()
          n451 = global write "Robot Global Data.vi" "RightBumper1"(FALSE ("RightBumper1")) -> ()
          n452 = global write "Robot Global Data.vi" "RightTrigger2"(0.0 ("RightTrigger2")) -> ()
          n453 = global write "Robot Global Data.vi" "LeftTrigger2"(1.0 ("LeftTrigger2")) -> ()
          n454 = global write "Robot Global Data.vi" "GyroReset"(TRUE ("RightBumper1")) -> ()
          n455 = global write "Robot Global Data.vi" "X1"(FALSE ("X1")) -> ()
          n456 = global write "Robot Global Data.vi" "LeftX1"(0.0 ("LeftX1")) -> ()
          n457 = global write "Robot Global Data.vi" "AutoState"("SpinUp" ("AutoState")) -> ()
          n458 = Wait (ms)(milliseconds to wait=u32 700) -> ()  [unwired: 1 out]
        }
        frame #4 {
          n459 = global write "Robot Global Data.vi" "RightBumper1"(FALSE ("RightBumper1")) -> ()
          n460 = global write "Robot Global Data.vi" "DriveENCreset"(FALSE ("RightBumper1")) -> ()
          n461 = global write "Robot Global Data.vi" "RightTrigger2"(1.0 ("RightTrigger2")) -> ()
          n462 = global write "Robot Global Data.vi" "LeftTrigger2"(1.0 ("LeftTrigger2")) -> ()
          n463 = global write "Robot Global Data.vi" "GyroReset"(FALSE ("RightBumper1")) -> ()
          n464 = global write "Robot Global Data.vi" "LeftX1"(0.0 ("LeftX1")) -> ()
          n465 = global write "Robot Global Data.vi" "X1"(FALSE ("X1")) -> ()
          n466 = global write "Robot Global Data.vi" "AutoState"("Shoot" ("AutoState")) -> ()
          n467 = Wait (ms)(milliseconds to wait=u32 1500) -> ()  [unwired: 1 out]
        }
        frame #5 {
          n468 = while {
            shift-right: [w517] -> _
            shift-left: _ -> [w532]
            shift-left: _ -> [w531]
            shift-left: _ -> [w530]
            shift-left: _ -> [w529]
            shift-left: _ -> [w533]
            shift-left: _ -> [w534]
            shift-left: _ -> [w528]
            shift-left: _ -> [w527]
            shift-left: _ -> [w526]
            shift-left: _ -> [w525]
            stop <- w520 stop-if-true
            n469 = Compound Arithmetic op=ADD(w534, w533, w532, w531, w530, w529, w528, w527, w526, w525) -> (w523:dbl)
            n470 = global read "Robot Global Data.vi" "Gyro Angle"() -> (w541:dbl)
            n471 = Wait (ms)(milliseconds to wait=u32 10) -> ()  [unwired: 1 out]
            n472 = Divide(x=w523, y=10.0) -> (x/y=w522:dbl)
            n473 = Absolute Value(x=w541) -> (abs(x)=w517:dbl)
            n474 = call "Elapsed Time4"() -> ("Time has Elapsed"=w519:bool)  [unwired: 12 in, 7 out]
            n475 = In Range and Coerce(upper limit=123.0, x=w522, lower limit=121.0) -> (In Range?=w538:bool)  [unwired: 1 out]
            n476 = call-poly <vilib>:"PID.vi"("output range"=cluster{"output high":dbl, "output low":dbl} {"output high"=0.6, "output low"=-0.6}, "PID gains"=T3 {"proportional gain (Kc)"=0.07, "integral time (Ti, min)"=0.0, "derivative time (Td, min)"=0.0}, "process variable"=w517, "setpoint"=122.0) -> ("output"=w535:dbl)  [unwired: 6 in, 1 out]
            n477 = Negate(x=w535) -> (-x=w518:dbl)
            n478 = Or(x=w538, y=w519) -> (x .or. y?=w520:bool)
            n479 = global write "Robot Global Data.vi" "LeftX1"(w518) -> ()
          }
          n480 = global write "Robot Global Data.vi" "RightBumper1"(FALSE ("RightBumper1")) -> ()
          n481 = global write "Robot Global Data.vi" "DriveENCreset"(FALSE ("RightBumper1")) -> ()
          n482 = global write "Robot Global Data.vi" "RightTrigger2"(0.0 ("RightTrigger2")) -> ()
          n483 = global write "Robot Global Data.vi" "LeftTrigger2"(0.0 ("LeftTrigger2")) -> ()
          n484 = global write "Robot Global Data.vi" "GyroReset"(FALSE ("RightBumper1")) -> ()
          n485 = global write "Robot Global Data.vi" "X1"(FALSE ("X1")) -> ()
          n486 = global write "Robot Global Data.vi" "AutoState"("Turn" ("AutoState")) -> ()
        }
        frame #6 {
          n487 = global write "Robot Global Data.vi" "DriveENCreset"(TRUE ("RightBumper1")) -> ()
          n488 = global write "Robot Global Data.vi" "RightBumper1"(FALSE ("RightBumper1")) -> ()
          n489 = global write "Robot Global Data.vi" "RightTrigger2"(0.0 ("RightTrigger2")) -> ()
          n490 = global write "Robot Global Data.vi" "LeftTrigger2"(0.0 ("LeftTrigger2")) -> ()
          n491 = global write "Robot Global Data.vi" "GyroReset"(TRUE ("RightBumper1")) -> ()
          n492 = global write "Robot Global Data.vi" "LeftX1"(0.0 ("LeftX1")) -> ()
          n493 = global write "Robot Global Data.vi" "X1"(FALSE ("X1")) -> ()
          n494 = global write "Robot Global Data.vi" "AutoState"("Reset" ("AutoState")) -> ()
          n495 = Wait (ms)(milliseconds to wait=u32 100) -> ()  [unwired: 1 out]
        }
        frame #7 {
          n496 = while {
            stop <- w559 stop-if-true
            n497 = Wait (ms)(milliseconds to wait=u32 10) -> ()  [unwired: 1 out]
            n498 = global read "Robot Global Data.vi" "RightEncAvg"() -> (w569:dbl)
            n499 = global read "Robot Global Data.vi" "LeftEncAvg"() -> (w568:dbl)
            n500 = Absolute Value(x=w569) -> (abs(x)=w562:dbl)
            n501 = Absolute Value(x=w568) -> (abs(x)=w561:dbl)
            n502 = Greater?(x=w562, y=110.0) -> (0:w566:bool)
            n503 = Greater?(x=w561, y=110.0) -> (0:w567:bool)
            n504 = And(x=w566, y=w567) -> (x .and. y?=w559:bool)
            n505 = Not(x=w559) -> (.not. x?=w563:bool)
            n506 = global write "Robot Global Data.vi" "RightBumper1"(w563) -> ()
          }
          n507 = global write "Robot Global Data.vi" "RightTrigger2"(0.0 ("RightTrigger2")) -> ()
          n508 = global write "Robot Global Data.vi" "DriveENCreset"(FALSE ("RightBumper1")) -> ()
          n509 = global write "Robot Global Data.vi" "LeftTrigger2"(0.0 ("LeftTrigger2")) -> ()
          n510 = global write "Robot Global Data.vi" "GyroReset"(FALSE ("RightBumper1")) -> ()
          n511 = global write "Robot Global Data.vi" "LeftX1"(0.0 ("LeftX1")) -> ()
          n512 = global write "Robot Global Data.vi" "X1"(TRUE ("X1")) -> ()
          n513 = global write "Robot Global Data.vi" "AutoState"("DriveForward2" ("AutoState")) -> ()
        }
        frame #8 {
          n514 = while {
            shift-right: [w577] -> _
            shift-left: _ -> [w591]
            shift-left: _ -> [w590]
            shift-left: _ -> [w589]
            shift-left: _ -> [w588]
            shift-left: _ -> [w592]
            shift-left: _ -> [w593]
            shift-left: _ -> [w587]
            shift-left: _ -> [w586]
            shift-left: _ -> [w585]
            shift-left: _ -> [w584]
            stop <- w579 stop-if-true
            n515 = Compound Arithmetic op=ADD(w593, w592, w591, w590, w589, w588, w587, w586, w585, w584) -> (w582:dbl)
            n516 = global read "Robot Global Data.vi" "Gyro Angle"() -> (w600:dbl)
            n517 = Wait (ms)(milliseconds to wait=u32 10) -> ()  [unwired: 1 out]
            n518 = Divide(x=w582, y=10.0) -> (x/y=w581:dbl)
            n519 = Absolute Value(x=w600) -> (abs(x)=w577:dbl)
            n520 = call "Elapsed Time5"() -> ("Time has Elapsed"=w578:bool)  [unwired: 12 in, 7 out]
            n521 = In Range and Coerce(upper limit=44.0, x=w581, lower limit=42.0) -> (In Range?=w597:bool)  [unwired: 1 out]
            n522 = call-poly <vilib>:"PID.vi"("output range"=cluster{"output high":dbl, "output low":dbl} {"output high"=0.6, "output low"=-0.6}, "PID gains"=T3 {"proportional gain (Kc)"=0.07, "integral time (Ti, min)"=0.0, "derivative time (Td, min)"=0.0}, "process variable"=w577, "setpoint"=43.0) -> ("output"=w594:dbl)  [unwired: 6 in, 1 out]
            n523 = Or(x=w597, y=w578) -> (x .or. y?=w579:bool)
            n524 = global write "Robot Global Data.vi" "LeftX1"(w594) -> ()
          }
          n525 = global write "Robot Global Data.vi" "RightBumper1"(FALSE ("RightBumper1")) -> ()
          n526 = global write "Robot Global Data.vi" "DriveENCreset"(FALSE ("RightBumper1")) -> ()
          n527 = global write "Robot Global Data.vi" "RightTrigger2"(0.0 ("RightTrigger2")) -> ()
          n528 = global write "Robot Global Data.vi" "LeftTrigger2"(0.0 ("LeftTrigger2")) -> ()
          n529 = global write "Robot Global Data.vi" "GyroReset"(FALSE ("RightBumper1")) -> ()
          n530 = global write "Robot Global Data.vi" "X1"(FALSE ("X1")) -> ()
          n531 = global write "Robot Global Data.vi" "AutoState"("Turn2" ("AutoState")) -> ()
        }
        frame #9 {
          n532 = global write "Robot Global Data.vi" "DriveENCreset"(FALSE ("RightBumper1")) -> ()
          n533 = global write "Robot Global Data.vi" "RightBumper1"(FALSE ("RightBumper1")) -> ()
          n534 = global write "Robot Global Data.vi" "RightTrigger2"(0.0 ("RightTrigger2")) -> ()
          n535 = global write "Robot Global Data.vi" "LeftTrigger2"(1.0 ("LeftTrigger2")) -> ()
          n536 = global write "Robot Global Data.vi" "GyroReset"(FALSE ("RightBumper1")) -> ()
          n537 = global write "Robot Global Data.vi" "X1"(FALSE ("X1")) -> ()
          n538 = global write "Robot Global Data.vi" "LeftX1"(0.0 ("LeftX1")) -> ()
          n539 = global write "Robot Global Data.vi" "AutoState"("SpinUp2" ("AutoState")) -> ()
          n540 = Wait (ms)(milliseconds to wait=u32 700) -> ()  [unwired: 1 out]
        }
        frame #10 {
          n541 = global write "Robot Global Data.vi" "RightBumper1"(FALSE ("RightBumper1")) -> ()
          n542 = global write "Robot Global Data.vi" "DriveENCreset"(FALSE ("RightBumper1")) -> ()
          n543 = global write "Robot Global Data.vi" "RightTrigger2"(1.0 ("RightTrigger2")) -> ()
          n544 = global write "Robot Global Data.vi" "LeftTrigger2"(1.0 ("LeftTrigger2")) -> ()
          n545 = global write "Robot Global Data.vi" "GyroReset"(FALSE ("RightBumper1")) -> ()
          n546 = global write "Robot Global Data.vi" "LeftX1"(0.0 ("LeftX1")) -> ()
          n547 = global write "Robot Global Data.vi" "X1"(FALSE ("X1")) -> ()
          n548 = global write "Robot Global Data.vi" "AutoState"("Shoot2" ("AutoState")) -> ()
          n549 = Wait (ms)(milliseconds to wait=u32 100) -> ()  [unwired: 1 out]
        }
        frame #11 {
          n550 = while {
            stop <- w627 stop-if-true
            n551 = Wait (ms)(milliseconds to wait=u32 10) -> ()  [unwired: 1 out]
            n552 = global read "Robot Global Data.vi" "RightEncAvg"() -> (w637:dbl)
            n553 = global read "Robot Global Data.vi" "LeftEncAvg"() -> (w636:dbl)
            n554 = Absolute Value(x=w637) -> (abs(x)=w630:dbl)
            n555 = Absolute Value(x=w636) -> (abs(x)=w629:dbl)
            n556 = Greater?(x=w630, y=160.0) -> (0:w634:bool)
            n557 = Greater?(x=w629, y=160.0) -> (0:w635:bool)
            n558 = And(x=w634, y=w635) -> (x .and. y?=w627:bool)
            n559 = Not(x=w627) -> (.not. x?=w631:bool)
            n560 = global write "Robot Global Data.vi" "RightBumper1"(w631) -> ()
          }
          n561 = global write "Robot Global Data.vi" "AutoState"("DriveForward3" ("AutoState")) -> ()
          n562 = global write "Robot Global Data.vi" "RightTrigger2"(0.0 ("RightTrigger2")) -> ()
          n563 = global write "Robot Global Data.vi" "DriveENCreset"(FALSE ("RightBumper1")) -> ()
          n564 = global write "Robot Global Data.vi" "LeftTrigger2"(0.0 ("LeftTrigger2")) -> ()
          n565 = global write "Robot Global Data.vi" "GyroReset"(FALSE ("RightBumper1")) -> ()
          n566 = global write "Robot Global Data.vi" "LeftX1"(0.0 ("LeftX1")) -> ()
          n567 = global write "Robot Global Data.vi" "X1"(TRUE ("X1")) -> ()
        }
        frame #12 {
          n568 = global write "Robot Global Data.vi" "DriveENCreset"(TRUE ("RightBumper1")) -> ()
          n569 = global write "Robot Global Data.vi" "RightBumper1"(FALSE ("RightBumper1")) -> ()
          n570 = global write "Robot Global Data.vi" "RightTrigger2"(0.0 ("RightTrigger2")) -> ()
          n571 = global write "Robot Global Data.vi" "LeftBumper1"(FALSE ("RightBumper1")) -> ()
          n572 = global write "Robot Global Data.vi" "LeftTrigger2"(0.0 ("LeftTrigger2")) -> ()
          n573 = global write "Robot Global Data.vi" "GyroReset"(FALSE ("RightBumper1")) -> ()
          n574 = global write "Robot Global Data.vi" "LeftX1"(0.0 ("LeftX1")) -> ()
          n575 = global write "Robot Global Data.vi" "X1"(TRUE ("X1")) -> ()
          n576 = global write "Robot Global Data.vi" "AutoState"("Intake pause" ("AutoState")) -> ()
          n577 = Wait (ms)(milliseconds to wait=u32 500) -> ()  [unwired: 1 out]
        }
        frame #13 {
          n578 = while {
            stop <- w655 stop-if-true
            n579 = Wait (ms)(milliseconds to wait=u32 10) -> ()  [unwired: 1 out]
            n580 = global read "Robot Global Data.vi" "RightEncAvg"() -> (w665:dbl)
            n581 = global read "Robot Global Data.vi" "LeftEncAvg"() -> (w664:dbl)
            n582 = Absolute Value(x=w665) -> (abs(x)=w658:dbl)
            n583 = Absolute Value(x=w664) -> (abs(x)=w657:dbl)
            n584 = Greater?(x=w658, y=60.0) -> (0:w662:bool)
            n585 = Greater?(x=w657, y=60.0) -> (0:w663:bool)
            n586 = And(x=w662, y=w663) -> (x .and. y?=w655:bool)
            n587 = Not(x=w655) -> (.not. x?=w659:bool)
            n588 = global write "Robot Global Data.vi" "LeftBumper1"(w659) -> ()
          }
          n589 = global write "Robot Global Data.vi" "AutoState"("DriveBack" ("AutoState")) -> ()
          n590 = global write "Robot Global Data.vi" "RightTrigger2"(0.0 ("RightTrigger2")) -> ()
          n591 = global write "Robot Global Data.vi" "DriveENCreset"(FALSE ("RightBumper1")) -> ()
          n592 = global write "Robot Global Data.vi" "LeftTrigger2"(0.0 ("LeftTrigger2")) -> ()
          n593 = global write "Robot Global Data.vi" "GyroReset"(FALSE ("RightBumper1")) -> ()
          n594 = global write "Robot Global Data.vi" "LeftX1"(0.0 ("LeftX1")) -> ()
          n595 = global write "Robot Global Data.vi" "X1"(TRUE ("X1")) -> ()
        }
        frame #14 {
          n596 = global write "Robot Global Data.vi" "DriveENCreset"(FALSE ("RightBumper1")) -> ()
          n597 = global write "Robot Global Data.vi" "RightBumper1"(FALSE ("RightBumper1")) -> ()
          n598 = global write "Robot Global Data.vi" "RightTrigger2"(0.0 ("RightTrigger2")) -> ()
          n599 = global write "Robot Global Data.vi" "LeftTrigger2"(1.0 ("LeftTrigger2")) -> ()
          n600 = global write "Robot Global Data.vi" "GyroReset"(FALSE ("RightBumper1")) -> ()
          n601 = global write "Robot Global Data.vi" "LeftBumper1"(FALSE ("RightBumper1")) -> ()
          n602 = global write "Robot Global Data.vi" "X1"(FALSE ("X1")) -> ()
          n603 = global write "Robot Global Data.vi" "LeftX1"(0.0 ("LeftX1")) -> ()
          n604 = global write "Robot Global Data.vi" "AutoState"("SpinUp3" ("AutoState")) -> ()
          n605 = Wait (ms)(milliseconds to wait=u32 700) -> ()  [unwired: 1 out]
        }
        frame #15 {
          n606 = global write "Robot Global Data.vi" "RightBumper1"(FALSE ("RightBumper1")) -> ()
          n607 = global write "Robot Global Data.vi" "DriveENCreset"(FALSE ("RightBumper1")) -> ()
          n608 = global write "Robot Global Data.vi" "RightTrigger2"(1.0 ("RightTrigger2")) -> ()
          n609 = global write "Robot Global Data.vi" "LeftTrigger2"(1.0 ("LeftTrigger2")) -> ()
          n610 = global write "Robot Global Data.vi" "GyroReset"(FALSE ("RightBumper1")) -> ()
          n611 = global write "Robot Global Data.vi" "LeftX1"(0.0 ("LeftX1")) -> ()
          n612 = global write "Robot Global Data.vi" "X1"(FALSE ("X1")) -> ()
          n613 = global write "Robot Global Data.vi" "AutoState"("Shoot3" ("AutoState")) -> ()
          n614 = Wait (ms)(milliseconds to wait=u32 3000) -> ()  [unwired: 1 out]
        }
        frame #16 {
          n615 = global write "Robot Global Data.vi" "RightBumper1"(FALSE ("RightBumper1")) -> ()
          n616 = global write "Robot Global Data.vi" "LeftTrigger2"(0.0 ("LeftTrigger2")) -> ()
          n617 = global write "Robot Global Data.vi" "RightTrigger2"(0.0 ("RightTrigger2")) -> ()
          n618 = global write "Robot Global Data.vi" "DriveENCreset"(FALSE ("RightBumper1")) -> ()
          n619 = global write "Robot Global Data.vi" "GyroReset"(FALSE ("RightBumper1")) -> ()
          n620 = global write "Robot Global Data.vi" "X1"(FALSE ("X1")) -> ()
          n621 = global write "Robot Global Data.vi" "AutoState"("Wait" ("AutoState")) -> ()
          n622 = Wait (ms)(milliseconds to wait=u32 10000) -> ()  [unwired: 1 out]
        }
      }
    }
    frame "Que3" {
      # "SetPoint\nDelay\nState"
      n623 = Bundle(0.0, "milliseconds to wait"=u32 10, "Initialize") -> (w743:cluster{dbl, "milliseconds to wait":u32, string})  [unwired: 1 in]
      n624 = Obtain Queue(max queue size (-1, unlimited)=-1, name (unnamed)="Autoque", element data type=w743) -> (queue out=w740:refnum<queue>)  [unwired: 2 in, 2 out]
      n625 = Flush Queue(queue=w740) -> (queue out=w736:refnum<queue>)  [unwired: 1 in, 2 out]
      n626 = Bundle(0.0, "milliseconds to wait"=u32 1000, "Intake") -> (w737:cluster{dbl, "milliseconds to wait":u32, string})  [unwired: 1 in]
      n627 = Enqueue Element(queue=w736, element=w737) -> (queue out=w735:refnum<queue>)  [unwired: 2 in, 2 out]
      n628 = Bundle(45.0, "milliseconds to wait"=u32 10, "Drive") -> (w732:cluster{dbl, "milliseconds to wait":u32, string})  [unwired: 1 in]
      n629 = Enqueue Element(queue=w735, element=w732) -> (queue out=w728:refnum<queue>)  [unwired: 2 in, 2 out]
      n630 = Bundle(0.0, "milliseconds to wait"=u32 10, "Shoot") -> (w729:cluster{dbl, "milliseconds to wait":u32, string})  [unwired: 1 in]
      n631 = Enqueue Element(queue=w728, element=w729) -> (queue out=w724:refnum<queue>)  [unwired: 2 in, 2 out]
      n632 = Bundle(90.0, "milliseconds to wait"=u32 10, "Turn") -> (w725:cluster{dbl, "milliseconds to wait":u32, string})  [unwired: 1 in]
      n633 = Enqueue Element(queue=w724, element=w725) -> (queue out=w720:refnum<queue>)  [unwired: 2 in, 2 out]
      n634 = Bundle(45.0, "milliseconds to wait"=u32 10, "Drive") -> (w721:cluster{dbl, "milliseconds to wait":u32, string})  [unwired: 1 in]
      n635 = Enqueue Element(queue=w720, element=w721) -> (queue out=w716:refnum<queue>)  [unwired: 2 in, 2 out]
      n636 = Bundle(113.0, "milliseconds to wait"=u32 10, "Turn") -> (w717:cluster{dbl, "milliseconds to wait":u32, string})  [unwired: 1 in]
      n637 = Enqueue Element(queue=w716, element=w717) -> (queue out=w712:refnum<queue>)  [unwired: 2 in, 2 out]
      n638 = Bundle(0.0, "milliseconds to wait"=u32 10, "Shoot") -> (w713:cluster{dbl, "milliseconds to wait":u32, string})  [unwired: 1 in]
      n639 = Enqueue Element(queue=w712, element=w713) -> (queue out=w708:refnum<queue>)  [unwired: 2 in, 2 out]
      n640 = Bundle(0.0, "milliseconds to wait"=u32 1000, "IntakeOff") -> (w709:cluster{dbl, "milliseconds to wait":u32, string})  [unwired: 1 in]
      n641 = Enqueue Element(queue=w708, element=w709) -> (queue out=w705:refnum<queue>)  [unwired: 2 in, 2 out]
      n642 = Bundle(0.0, "milliseconds to wait"=u32 100, "Stop") -> (w693:cluster{dbl, "milliseconds to wait":u32, string})  [unwired: 1 in]
      n643 = Enqueue Element(queue=w705, element=w693) -> (queue out=w704:refnum<queue>)  [unwired: 2 in, 2 out]
      n644 = while {
        shift-right: [w753] -> _
        shift-left: w704 -> [w756]
        stop <- FALSE stop-if-true
        # "Publish Current\nState To Dashboard"
        n645 = Preview Queue Element(queue=w756) -> (queue out=w755:refnum<queue>, element=w754:cluster{dbl, "milliseconds to wait":u32, string})  [unwired: 2 in, 2 out]
        n646 = Unbundle(w754) -> (w752:dbl, w747:string)  [unwired: 1 out]
        "Current action" <- w747
        n647 = global write "Robot Global Data.vi" "POV1"(i16 -1 ("POV1")) -> ()
        n648 = global write "Robot Global Data.vi" "POV2"(i16 -1 ("POV2")) -> ()
        n649 = global read "Robot Global Data.vi" "Gyro Angle"() -> (w751:dbl)
        n650 = Absolute Value(x=w751) -> (abs(x)=w746:dbl)
        n651 = case shown="\"Turning\"" w747 {
          tunnel: w755 -> [w764 w775 w787 w795 w808 w824 w832 w842 w854 w862 w877 w878]
          tunnel: [w760 w773 w778 w789 w801 w810 w829 w835 w851 w861 w876 w878] -> w753
          tunnel: w752 -> [_ _ _ _ _ _ _ _ _ w860 _ _]
          tunnel: w746 -> [_ _ _ _ _ _ _ _ _ w856 _ _]
          frame "Default", Default {
            n652 = Dequeue Element(queue=w764) -> (queue out=w760:refnum<queue>, element=w763:cluster{dbl, "milliseconds to wait":u32, string})  [unwired: 2 in, 2 out]
            n653 = Unbundle(w763) -> ("milliseconds to wait"=w762:u32)  [unwired: 2 out]
            n654 = Wait (ms)(milliseconds to wait=w762) -> ()  [unwired: 1 out]
            n655 = global write "Robot Global Data.vi" "RightTrigger2"(0.0 ("RightTrigger2")) -> ()
            n656 = global write "Robot Global Data.vi" "LeftX1"(0.0 ("LeftX1")) -> ()
          }
          frame "Intake" {
            n657 = Dequeue Element(queue=w775) -> (queue out=w773:refnum<queue>, element=w777:cluster{dbl, "milliseconds to wait":u32, string})  [unwired: 2 in, 2 out]
            n658 = Unbundle(w777) -> ("milliseconds to wait"=w776:u32)  [unwired: 2 out]
            n659 = Wait (ms)(milliseconds to wait=w776) -> ()  [unwired: 1 out]
            n660 = global write "Robot Global Data.vi" "DriveENCreset"(TRUE ("RightBumper1")) -> ()
            n661 = global write "Robot Global Data.vi" "RightBumper1"(FALSE ("RightBumper1")) -> ()
            n662 = global write "Robot Global Data.vi" "RightTrigger2"(0.0 ("RightTrigger2")) -> ()
            n663 = global write "Robot Global Data.vi" "LeftTrigger2"(0.0 ("LeftTrigger2")) -> ()
            n664 = global write "Robot Global Data.vi" "GyroReset"(TRUE ("RightBumper1")) -> ()
            n665 = global write "Robot Global Data.vi" "LeftX1"(0.0 ("LeftX1")) -> ()
            n666 = global write "Robot Global Data.vi" "X1"(FALSE ("X1")) -> ()
            n667 = global write "Robot Global Data.vi" "X1"(TRUE ("X1")) -> ()
            n668 = global write "Robot Global Data.vi" "LeftX1"(0.0 ("LeftX1")) -> ()
          }
          frame "Drive" {
            n669 = Dequeue Element(queue=w787) -> (queue out=w780:refnum<queue>, element=w788:cluster{dbl, "milliseconds to wait":u32, string})  [unwired: 2 in, 2 out]
            n670 = Unbundle(w788) -> (w786:dbl, "milliseconds to wait"=w779:u32)  [unwired: 1 out]
            n671 = global read "Robot Global Data.vi" "LeftEncAvg"() -> (w785:dbl)
            n672 = Wait (ms)(milliseconds to wait=w779) -> ()  [unwired: 1 out]
            n673 = Add(x=w786, y=w785) -> (x+y=w784:dbl)
            n674 = Bundle(w784, "milliseconds to wait"=u32 10, "Driving") -> (w781:cluster{dbl, "milliseconds to wait":u32, string})  [unwired: 1 in]
            n675 = Enqueue Element At Opposite End(queue=w780, element=w781) -> (queue out=w778:refnum<queue>)  [unwired: 2 in, 2 out]
          }
          frame "Driving" {
            n676 = Preview Queue Element(queue=w795) -> (queue out=w791:refnum<queue>, element=w794:cluster{dbl, "milliseconds to wait":u32, string})  [unwired: 2 in, 2 out]
            n677 = Unbundle(w794) -> (w793:dbl)  [unwired: 2 out]
            n678 = global read "Robot Global Data.vi" "LeftEncAvg"() -> (w792:dbl)
            n679 = Less Or Equal?(x=w792, y=w793) -> (x <= y?=w790:bool)
            n680 = case shown="True" w790 {
              tunnel: w791 -> [w797 w800]
              tunnel: [w796 w800] -> w789
              frame False {
                n681 = global write "Robot Global Data.vi" "RightTrigger1"(0.0 ("RightTrigger1")) -> ()
                n682 = Dequeue Element(queue=w797) -> (queue out=w796:refnum<queue>)  [unwired: 2 in, 3 out]
              }
              frame True {
                n683 = global write "Robot Global Data.vi" "RightTrigger1"(0.75 ("RightTrigger1")) -> ()
              }
            }
          }
          frame "Shoot" {
            n684 = Dequeue Element(queue=w808) -> (queue out=w804:refnum<queue>, element=w809:cluster{dbl, "milliseconds to wait":u32, string})  [unwired: 2 in, 2 out]
            n685 = Unbundle(w809) -> (w803:dbl, "milliseconds to wait"=w807:u32)  [unwired: 1 out]
            n686 = Wait (ms)(milliseconds to wait=w807) -> ()  [unwired: 1 out]
            n687 = Bundle(w803, "milliseconds to wait"=u32 200, "SpinUp") -> (w802:cluster{dbl, "milliseconds to wait":u32, string})  [unwired: 1 in]
            n688 = Enqueue Element At Opposite End(queue=w804, element=w802) -> (queue out=w801:refnum<queue>)  [unwired: 2 in, 2 out]
          }
          frame "SpinUp" {
            n689 = Dequeue Element(queue=w824) -> (queue out=w822:refnum<queue>, element=w821:cluster{dbl, "milliseconds to wait":u32, string})  [unwired: 2 in, 2 out]
            n690 = Wait (ms)(milliseconds to wait=u32 10) -> ()  [unwired: 1 out]
            n691 = Unbundle(w821) -> (w820:dbl, "milliseconds to wait"=w819:u32)  [unwired: 1 out]
            n692 = Decrement(x=w819) -> (x-1=w816:u32)
            n693 = global write "Robot Global Data.vi" "LeftTrigger2"(1.0 ("LeftTrigger2")) -> ()
            n694 = Equal?(x=w816, y=u32 0) -> (x = y?=w817:bool)
            n695 = Select(t="KickUp", s=w817, f="SpinUp") -> (s? t:f=w812:string)
            n696 = Bundle(w820, w816, w812) -> (w815:cluster{dbl, u32, string})  [unwired: 1 in]
            n697 = Enqueue Element At Opposite End(queue=w822, element=w815) -> (queue out=w810:refnum<queue>)  [unwired: 2 in, 2 out]
          }
          frame "KickUp" {
            n698 = Dequeue Element(queue=w832) -> (queue out=w830:refnum<queue>, element=w831:cluster{dbl, "milliseconds to wait":u32, string})  [unwired: 2 in, 2 out]
            n699 = Wait (ms)(milliseconds to wait=u32 1000) -> ()  [unwired: 1 out]
            n700 = Unbundle(w831) -> (w828:dbl)  [unwired: 2 out]
            n701 = Bundle(w828, "milliseconds to wait"=u32 50, "Name"="ShootOff") -> (w827:T4)  [unwired: 1 in]
            n702 = Enqueue Element At Opposite End(queue=w830, element=w827) -> (queue out=w829:refnum<queue>)  [unwired: 2 in, 2 out]
            n703 = global write "Robot Global Data.vi" "RightTrigger2"(1.0 ("RightTrigger2")) -> ()
          }
          frame "ShootOff" {
            n704 = Wait (ms)(milliseconds to wait=u32 50) -> ()  [unwired: 1 out]
            n705 = Dequeue Element(queue=w842) -> (queue out=w837:refnum<queue>, element=w838:cluster{dbl, "milliseconds to wait":u32, string})  [unwired: 2 in, 2 out]
            n706 = Unbundle(w838) -> (w841:dbl)  [unwired: 2 out]
            n707 = Bundle(w841, "milliseconds to wait"=u32 10, "Null") -> (w836:cluster{dbl, "milliseconds to wait":u32, string})  [unwired: 1 in]
            n708 = Enqueue Element At Opposite End(queue=w837, element=w836) -> (queue out=w835:refnum<queue>)  [unwired: 2 in, 2 out]
            n709 = global write "Robot Global Data.vi" "RightTrigger2"(0.0 ("RightTrigger2")) -> ()
          }
          frame "Turn" {
            n710 = Dequeue Element(queue=w854) -> (queue out=w852:refnum<queue>, element=w850:cluster{dbl, "milliseconds to wait":u32, string})  [unwired: 2 in, 2 out]
            n711 = global write "Robot Global Data.vi" "GyroReset"(TRUE ("GyroReset")) -> ()
            n712 = global write "Robot Global Data.vi" "RightTrigger2"(0.0 ("RightTrigger2")) -> ()
            n713 = Unbundle(w850) -> (w849:dbl, "milliseconds to wait"=w848:u32)  [unwired: 1 out]
            n714 = Bundle(w849, "milliseconds to wait"=w848, "Name"="Turning") -> (w846:T4)  [unwired: 1 in]
            n715 = Enqueue Element At Opposite End(queue=w852, element=w846) -> (queue out=w851:refnum<queue>)  [unwired: 2 in, 2 out]
          }
          frame "Turning" {
            n716 = Decrement(x=w860) -> (x-1=w858:dbl)
            n717 = Increment(x=w860) -> (x+1=w859:dbl)
            n718 = In Range and Coerce(upper limit=w859, x=w856, lower limit=w858) -> (In Range?=w857:bool)  [unwired: 1 out]
            n719 = global write "Robot Global Data.vi" "GyroReset"(FALSE ("GyroReset")) -> ()
            n720 = case shown="False" w857 {
              tunnel: w860 -> [w865 _]
              tunnel: w856 -> [w864 _]
              tunnel: w862 -> [w863 w871]
              tunnel: [w863 w870] -> w861
              frame False {
                n721 = call-poly <vilib>:"PID.vi"("output range"=cluster{"output high":dbl, "output low":dbl} {"output high"=0.7, "output low"=-0.7}, "PID gains"=T3 {"proportional gain (Kc)"=0.05, "integral time (Ti, min)"=0.0, "derivative time (Td, min)"=0.0}, "process variable"=w864, "setpoint"=w865) -> ("output"=w868:dbl)  [unwired: 6 in, 1 out]
                n722 = Negate(x=w868) -> (-x=w867:dbl)
                n723 = global write "Robot Global Data.vi" "LeftX1"(w867) -> ()
              }
              frame True {
                n724 = global write "Robot Global Data.vi" "LeftX1"(0.0 ("LeftX1")) -> ()
                n725 = Dequeue Element(queue=w871) -> (queue out=w870:refnum<queue>)  [unwired: 2 in, 3 out]
              }
            }
          }
          frame "IntakeOff" {
            n726 = Dequeue Element(queue=w877) -> (queue out=w876:refnum<queue>, element=w875:cluster{dbl, "milliseconds to wait":u32, string})  [unwired: 2 in, 2 out]
            n727 = Unbundle(w875) -> ("milliseconds to wait"=w874:u32)  [unwired: 2 out]
            n728 = Wait (ms)(milliseconds to wait=w874) -> ()  [unwired: 1 out]
            n729 = global write "Robot Global Data.vi" "X1"(TRUE ("X1")) -> ()
          }
          frame "Stop" {
          }
        }
        n730 = Wait (ms)(milliseconds to wait=u32 10) -> ()  [unwired: 1 out]
        n731 = call-poly <vilib>:"NT Write Value.vi"("String"=w747, "Name"="DB/String 9") -> ()  [unwired: 9 in, 1 out]
      }
    }
  }
